vi "Washer DOE SM.vi"() -> ()   [LabVIEW 2012]
uses:
  Nufi/subVI/States.ctl
  Nufi/subVI/Data.ctl
  Nufi/subVI/logData.ctl
  C:/Users/220038920/Desktop/CVS Folder/NI-2010/Trunk/Washer DOE/Portable Stand/Nufi/dll/GeaCommunication.dll
  Nufi/dll/GeaCommunication.dll
  Nufi/subVI/Nufi Global_ReceivedDataCluster.vi
  <vilib>/Utility/file.llb/Read From Spreadsheet File (string).vi
panel:
  out "Model Information":string[][](array[string])
  out "Elapsed Time (sec)":dbl format="%.2f"
  out "Current State":string
  in  "First Time Through":bool=TRUE
  out "error out":errorcluster
  in  "Total Gallons Hot":dbl
  in  "Total Gallons Cold":dbl
  out "Loop Time":dbl
  in  "FrontPanel Meters 2":T1
  in  "Tab Control":enum32{"Test Screen", "Raw Data"}(tab)
  in  "Tab Control 3":T2(tab)
  in  "Initial Cloth Weight":dbl
  out "Enter File Init State":bool
  out "All Fields Complete":bool
  in  "Agitator:":u16(ring) items=["", "YES", "NO"]
  in  "File Setup OK":bool
  in  "Comments:":string
  in  "Voltage:":dbl
  in  "Water Pressure:":dbl
  in  "Cycle Selection:":string
  in  "Cold Water Temperature (Fahrenheit):":string
  in  "Hot Water Temperature (Fahrenheit):":string
  in  "Cloth Lot:":string
  in  "Capacity (cu.ft):":dbl
  in  "Hot Rinse Available:":u16(ring)
  in  "Extra Hot Wash Available:":u16(ring)
  in  "Number of Warm Washes:":dbl
  in  "Fill Method:":string
  in  "Station ID:":u16(ring) items=["", "Station 1", "Station 2", "Station 3", "Station 4", "Station 5", "Station 6", "Station 7", "Station 8", ""]
  in  "Lab ID:":string
  out "Test Date:":timestamp
  in  "Serial Number:":string
  in  "Model Number:":string
  in  "Engineer:":string
  in  "Technician:":string
  in  "Engineering ID:":string
  in  "Special Notes:":string
  out "File Path":path
  out "Complete?":bool
  in  "Update Button":bool
  in  "Manual Fill":bool
  in  "Coin Op":bool
  in  "Hawk":bool
  in  "Viper":bool
  in  "Complete DOE Cap":bool
  in  "Washer 4":T3
  in  "Washer 3":T4
  in  "Washer 2":T5
  in  "Washer 1":T6
  out "Test Date:DOE Cap":timestamp caption="Test Date:"
  out "Technician:DOE Cap":string caption="Technician:"
  in  "Command:Data":string caption="Debug Log"
  in  "Clear":bool
  in  "StartLog":bool
  in  "Path":bool
  out "UI Version":string
  out "Param. Ver.":string
  out "Personality":string
  in  "recirc":bool
  out "Recirc":bool
  in  "drain":bool
  out "Drain":bool
  in  "fs":bool
  out "FS":bool
  in  "det":bool
  out "Det":bool
  in  "cold":bool
  out "Cold":bool
  in  "hot":bool
  out "Hot":bool
  in  "Viper/Hawk":u16(ring) items=["Viper", "Hawk"]
  in  "Source":u8=228 format="%x"
  in  "Address":u8=35 format="%x"
  out "GEA2":bool
  out "Board ID":string
  out "Lid Closed?":bool
  out "Lid Locked?":bool
  out "FrontPanel Meters":T7 {"Rinse Hot" format="%#.3g"; "Rinse Cold" format="%#.3g"; "Hot Water Total During Wash" format="%#.3g"; "Cold Water Total During Wash" format="%#.3g"; "Volts" format="%#.3g"; "Current" format="%#.3g"; "Watts" format="%#.3g"; "Watt Hour" format="%#.3g"; "Hot Water Total" format="%#.3g"; "Hot Water Rate" format="%#.3g"; "Cold Water Total" format="%#.3g"; "Cold Water Rate" format="%#.3g"; "Hot Water Pressure" format="%#.3g"; "Hot Water Temperature" format="%#.3g"; "Cold Water Pressure" format="%#.3g"; "Cold Water Temperature" format="%#.3g"}
  out "Fabric Softener":u32
  out "Detergent":u32
  out "Speed":u32
  out "Load Size":u32
  out "Direction":string
  out "Temperature":u8
  out "Water Pressure":u32
  in  "Off Mode Watts":dbl
  in  "Standby Mode Watts":dbl
  out "Elapsed Time":dbl format="%<%H:%M:%S>t"
  in  "Tab Control 4":enum32{"Watts", "Control Settings"}(tab)
  out "Recirc 3":dbl(graph)
  out "Incoder Position":string
  out "Pre Soak":string
  out "Spin Setting":string
  out "Temperature Setting":string
  out "Soil Setting":string
  out "Total Gallons Used":string
  in  "Stop":bool
  in  "Start":bool
  in  "Reset All":bool
  out "Array":string[][](array[string])
  in  "DOE Capacity Path":path=path "C:/GE/Washer DOE/DOE Capacity.txt"
  in  "Calibration File Path":path=path "C:/Program Files/GE/Washer DOE/CalibrationDates.txt"
  in  "VISA Laurel Meter":refnum<visa-resource-name>="LaurelMeter"
  in  "Aplus IP Address":string="192.168.1.101"
  in  "Remote Port":i32=502
  out "Start Time (sec)":dbl format="%<%H:%M:%S>t"
  in  "Send":bool
  in  "Data":u8[](array[numeric]) format="%.0x"
  in  "Command":u8 format="%.0x"
  in  "Exit":bool
  in  "EOL":bool
  in  "2015?":bool
  in  "Low Power Switch":bool
  in  "SaveGraph":bool
  in  "All Models Excel Sheet":path=path "C:/GE/Washer DOE"
  in  "Network Model Location":path=path "\\\\3.67.38.12\\share/Test Data/Washer DOE/Models"
  # "Take the Family, Model, and Capacity."
  # "Test Conditions"
  # "Model Details"
  # "DOE Capacity Measurements Per 10 CFR 430 Appendix J1"
  # "Standard Values"
  # "Measured\nTemp (Deg F)"
  # "Weigh of \nWater (lbs)"
  # "Model Number"
  # "Serial Number"
  # "Lab Number"
  # "This will only update at the end of the cycle"
  # "x"
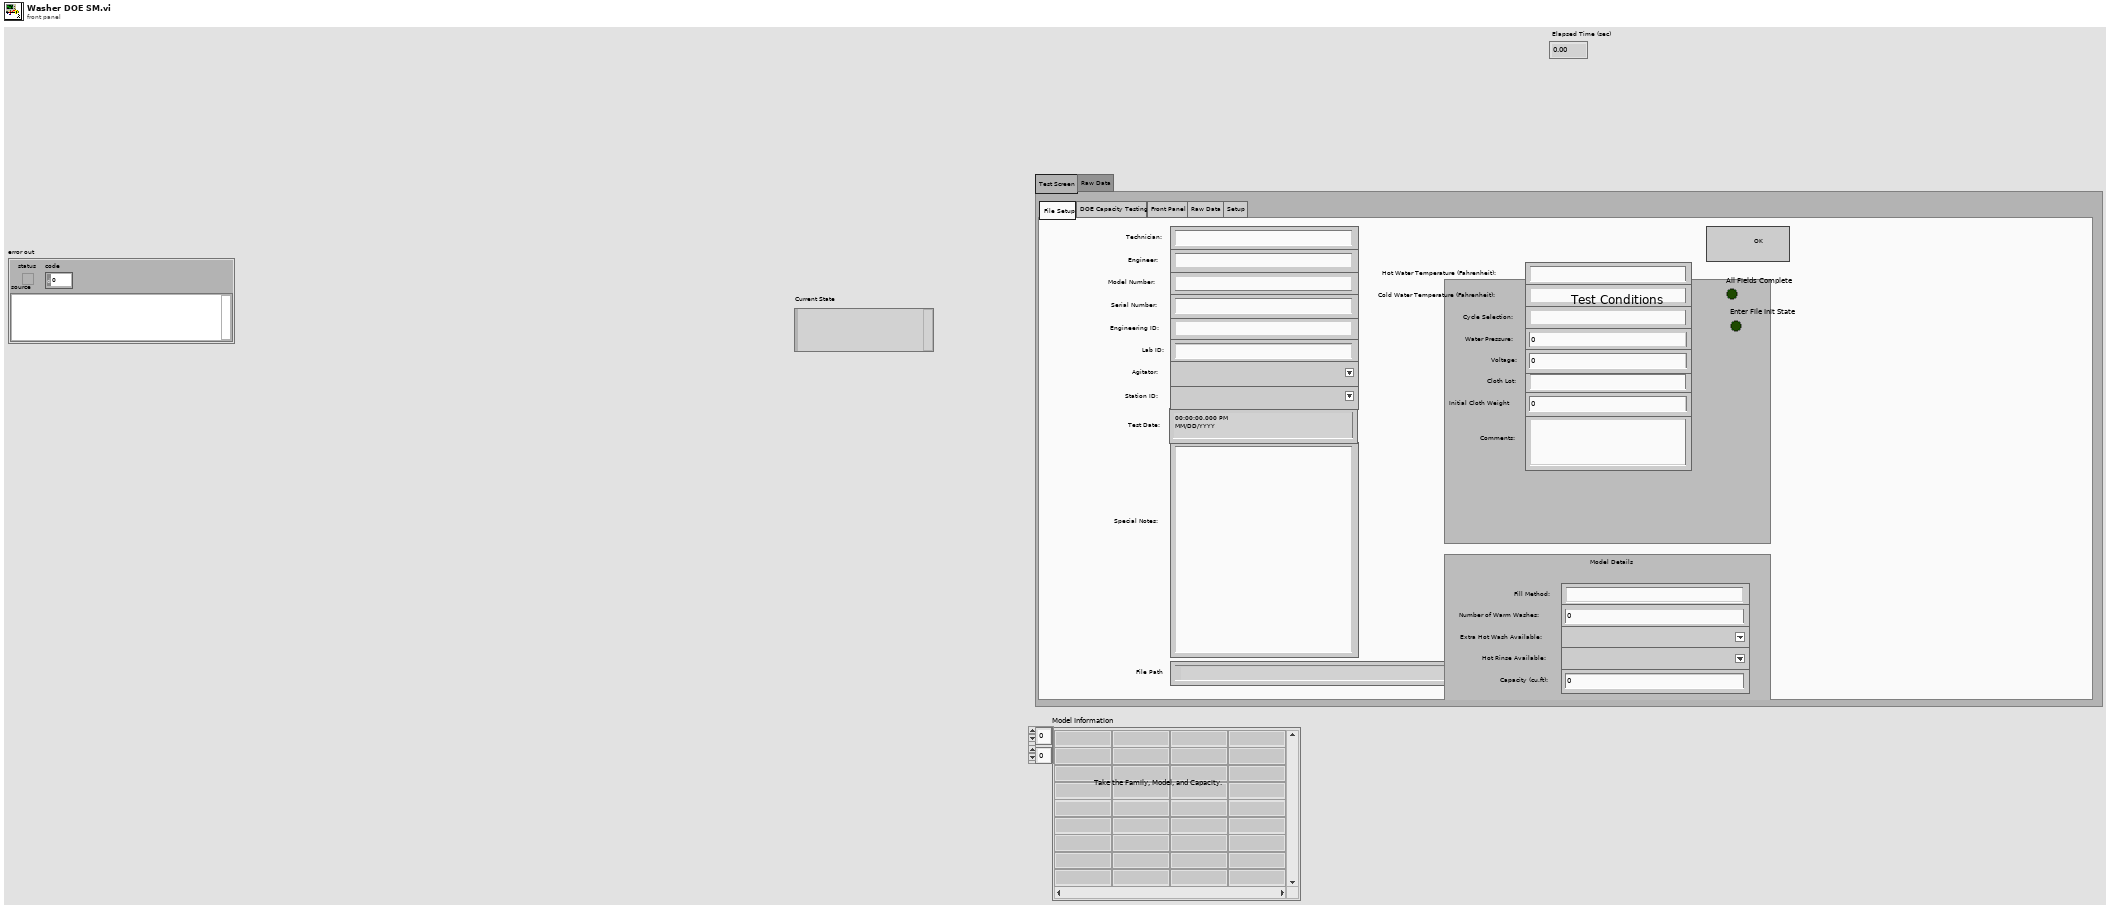
[diagram p1: front panel]
types:
  T1 = cluster{"Cold Water\nTemperature":dbl, "Cold Water\nPressure":dbl, "Hot Water\nTemperature":dbl, "Hot Water\nPressure":dbl, "Cold Water\nRate":dbl, "Cold Water\nTotal":dbl, "Hot Water\n Rate":dbl, "Hot Water\nTotal":dbl, "Watt Hour":dbl, "Watts":dbl, "Current":dbl, "Volts":dbl, "Cold Water Total During Wash":dbl, "Hot Water Total During Wash":dbl, "Rinse Cold":dbl, "Rinse Hot":dbl}
  T2 = enum32{"File Setup", "DOE Capacity Testing", "Front Panel", "Raw Data", "Setup"}
  T3 = cluster{"Measured Temp (Deg F)3":dbl, "Weight of Water (lbs)3":dbl, "Lab Number3":string, "Serial Number3":string, "Model Number3":string}
  T4 = cluster{"Measured Temp (Deg F)2":dbl, "Weight of Water (lbs)2":dbl, "Lab Number2":string, "Serial Number2":string, "Model Number2":string}
  T5 = cluster{"Measured Temp (Deg F )1":dbl, "Weight of Water (lbs)1":dbl, "Lab Number1":string, "Serial Number1":string, "Model Number1":string}
  T6 = cluster{"Measured Temp":dbl, "Water Weight":dbl, "Lab Number":string, "Serial Number":string, "Model Number":string}
  T7 = cluster{"Cold Water Temperature":dbl, "Cold Water Pressure":dbl, "Hot Water Temperature":dbl, "Hot Water Pressure":dbl, "Cold Water Rate":dbl, "Cold Water Total":dbl, "Hot Water Rate":dbl, "Hot Water Total":dbl, "Watt Hour":dbl, "Watts":dbl, "Current":dbl, "Volts":dbl, "Cold Water Total During Wash":dbl, "Hot Water Total During Wash":dbl, "Rinse Cold":dbl, "Rinse Hot":dbl}
  T8 = typedef "Data.ctl" = cluster{"GEA2 Message Ref":refnum<k24>, "Board ID":string, "USB Connect":refnum<k24>, "GEA Bus":refnum<k24>, "Address":u8, "Source":u8, "Message Count":dbl, "ReceivedData":u8[], "Log?":bool, "Partial Message String":string, "Full Message to Save":string, "Data to send":u8[], "Command":u8, "selected path":path, "debugRef":refnum<file>, "dataRef":refnum<file>, "logData":T9, "GraphData":T9[]}
  T9 = typedef "logData.ctl" = cluster{"IGBT Temp":u8, "Speed":u32, "Load Size":u32, "Temperature":u8, "Water Pressure":u32, "Detergent":u32, "Fabric Softener":u32, "Direction":string, "Det":bool, "FS":bool, "Recirc":bool, "Drain":bool, "Hot":bool, "Cold":bool, "LidClosed":bool, "LidLocked":bool}
  T10 = typedef "States.ctl" = enum16{"-------- Initialize --------", "Data", "GEA2", "---------- Core ----------", "Wait", "Read Debug", "Read MC Data", "Read Inv Data", "Read Incoder Position", "Read LEDs", "Update Graphs", "Send CMD", "Log Debug", "Log Data", "Test", "Exit"}
  T11 = enum8{"Enabled", "Disabled", "Disabled and Grayed Out"}
  T12 = typedef "Nufi Message.ctl" = cluster{"ReceivedData":u8[], "Count":dbl, "Source Address":u8, "Destination Addresss":u8, "Command":u8, "Days":i32, "Hours":i32, "Minutes":i32, "Seconds":i32, "Milliseconds":i32}
  T13 = enum16{"open", "replace", "create", "open or create", "replace or create", "replace or create with confirmation"}
  T14 = cluster{"IGBT Temp":bool, "Speed":bool, "Load Size":bool, "Temperature":bool, "Water Pressure":bool, "Detergent":bool, "Fabric Softener":bool, "Direction":bool, "Det":bool, "FS":bool, "Recirc":bool, "Drain":bool, "Hot":bool, "Cold":bool, "LidClosed":bool, "LidLocked":bool}
  T15 = enum32{"invalid app kind", "Development System", "Run Time System", "Student Edition", "Embedded LabVIEW", "Evaluation", "Custom"}
  T16 = enum16{"Command Mode", "Cold Reset", "Function Reset", "Reading: All Active Items", "Reading: Item 1", "Reading: Item 2", "Reading: Item 3"}
  T17 = enum32{"Invalid", "Standard", "Closed", "Hidden", "Minimized", "Maximized"}
  T18 = cluster{"Measured Temp":dbl, "Weight of Water":dbl, "Lab Number":string, "Serial Number":string, "Model Number":string}
  T19 = cluster{"Core":cluster{"Current VI Reference":refnum<vi>, "Close Panel on Exit?":bool}, "Remote Port":i32, "Aplus IP Address":string, "Power":cluster{"Voltage":sgl, "Current":sgl, "Frequency":sgl, "Power":sgl, "Power Factor":sgl}, "Watt Hours":dbl, "Total Array":dbl[], "VISA Laurel Meter":refnum<visa-resource-name>, "FrontPanel Meters 2":cluster{"Cold Water\nTemperature":dbl, "Cold Water\nPressure":dbl, "Hot Water\nTemperature":dbl, "Hot Water\nPressure":dbl, "Cold Water\nRate":dbl, "Cold Water\nTotal":dbl, "Hot Water\n Rate":dbl, "Hot Water\nTotal":dbl, "Watt Hour":dbl, "Watts":dbl, "Current":dbl, "Volts":dbl, "Cold Water Total During Wash":dbl, "Hot Water Total During Wash":dbl, "Rinse Cold":dbl, "Rinse Hot":dbl}, "Total Gallons Cold":dbl, "Total Gallons Hot":dbl, "2015?":bool, "Off Mode Watts":dbl, "Standby Mode Watts":dbl, "Low Power Switch":bool, "First Time Through":bool, "Calibration":string[][], "Washer 1":cluster{"Measured Temp":dbl, "Water Weight":dbl, "Lab Number":string, "Serial Number":string, "Model Number":string}, "Washer 2":cluster{"Measured Temp (Deg F )1":dbl, "Weight of Water (lbs)1":dbl, "Lab Number1":string, "Serial Number1":string, "Model Number1":string}, "Washer 3":cluster{"Measured Temp (Deg F)2":dbl, "Weight of Water (lbs)2":dbl, "Lab Number2":string, "Serial Number2":string, "Model Number2":string}, "Washer 4":cluster{"Measured Temp (Deg F)3":dbl, "Weight of Water (lbs)3":dbl, "Lab Number3":string, "Serial Number3":string, "Model Number3":string}, cluster{"Calibration File Path":path, "DOE Capacity Path":path, "All Models Excel Sheet":path, "Network Model Location":path}, "Complete DOE Cap":bool}
  T20 = cluster{"Calibration File Path":path, "DOE Capacity Path":path, "All Models Excel Sheet":path, "Network Model Location":path}
  T21 = cluster{"Voltage":sgl, "Current":sgl, "Frequency":sgl, "Power":sgl, "Power Factor":sgl}
  T22 = cluster{"Current VI Reference":refnum<vi>, "Close Panel on Exit?":bool}
  T23 = cluster{"Cold Water Pressure":dbl, "Hot Water Pressure":dbl, "Cold Water Temp":dbl, "Hot Water Temp":dbl, "Ambient Temp":dbl, "Room Humidity":dbl}
  T24 = cluster{"Voltage":sgl, "Current":sgl, "Frequency":sgl, "Power":sgl, "Power Factor":sgl, "WattHours":sgl}
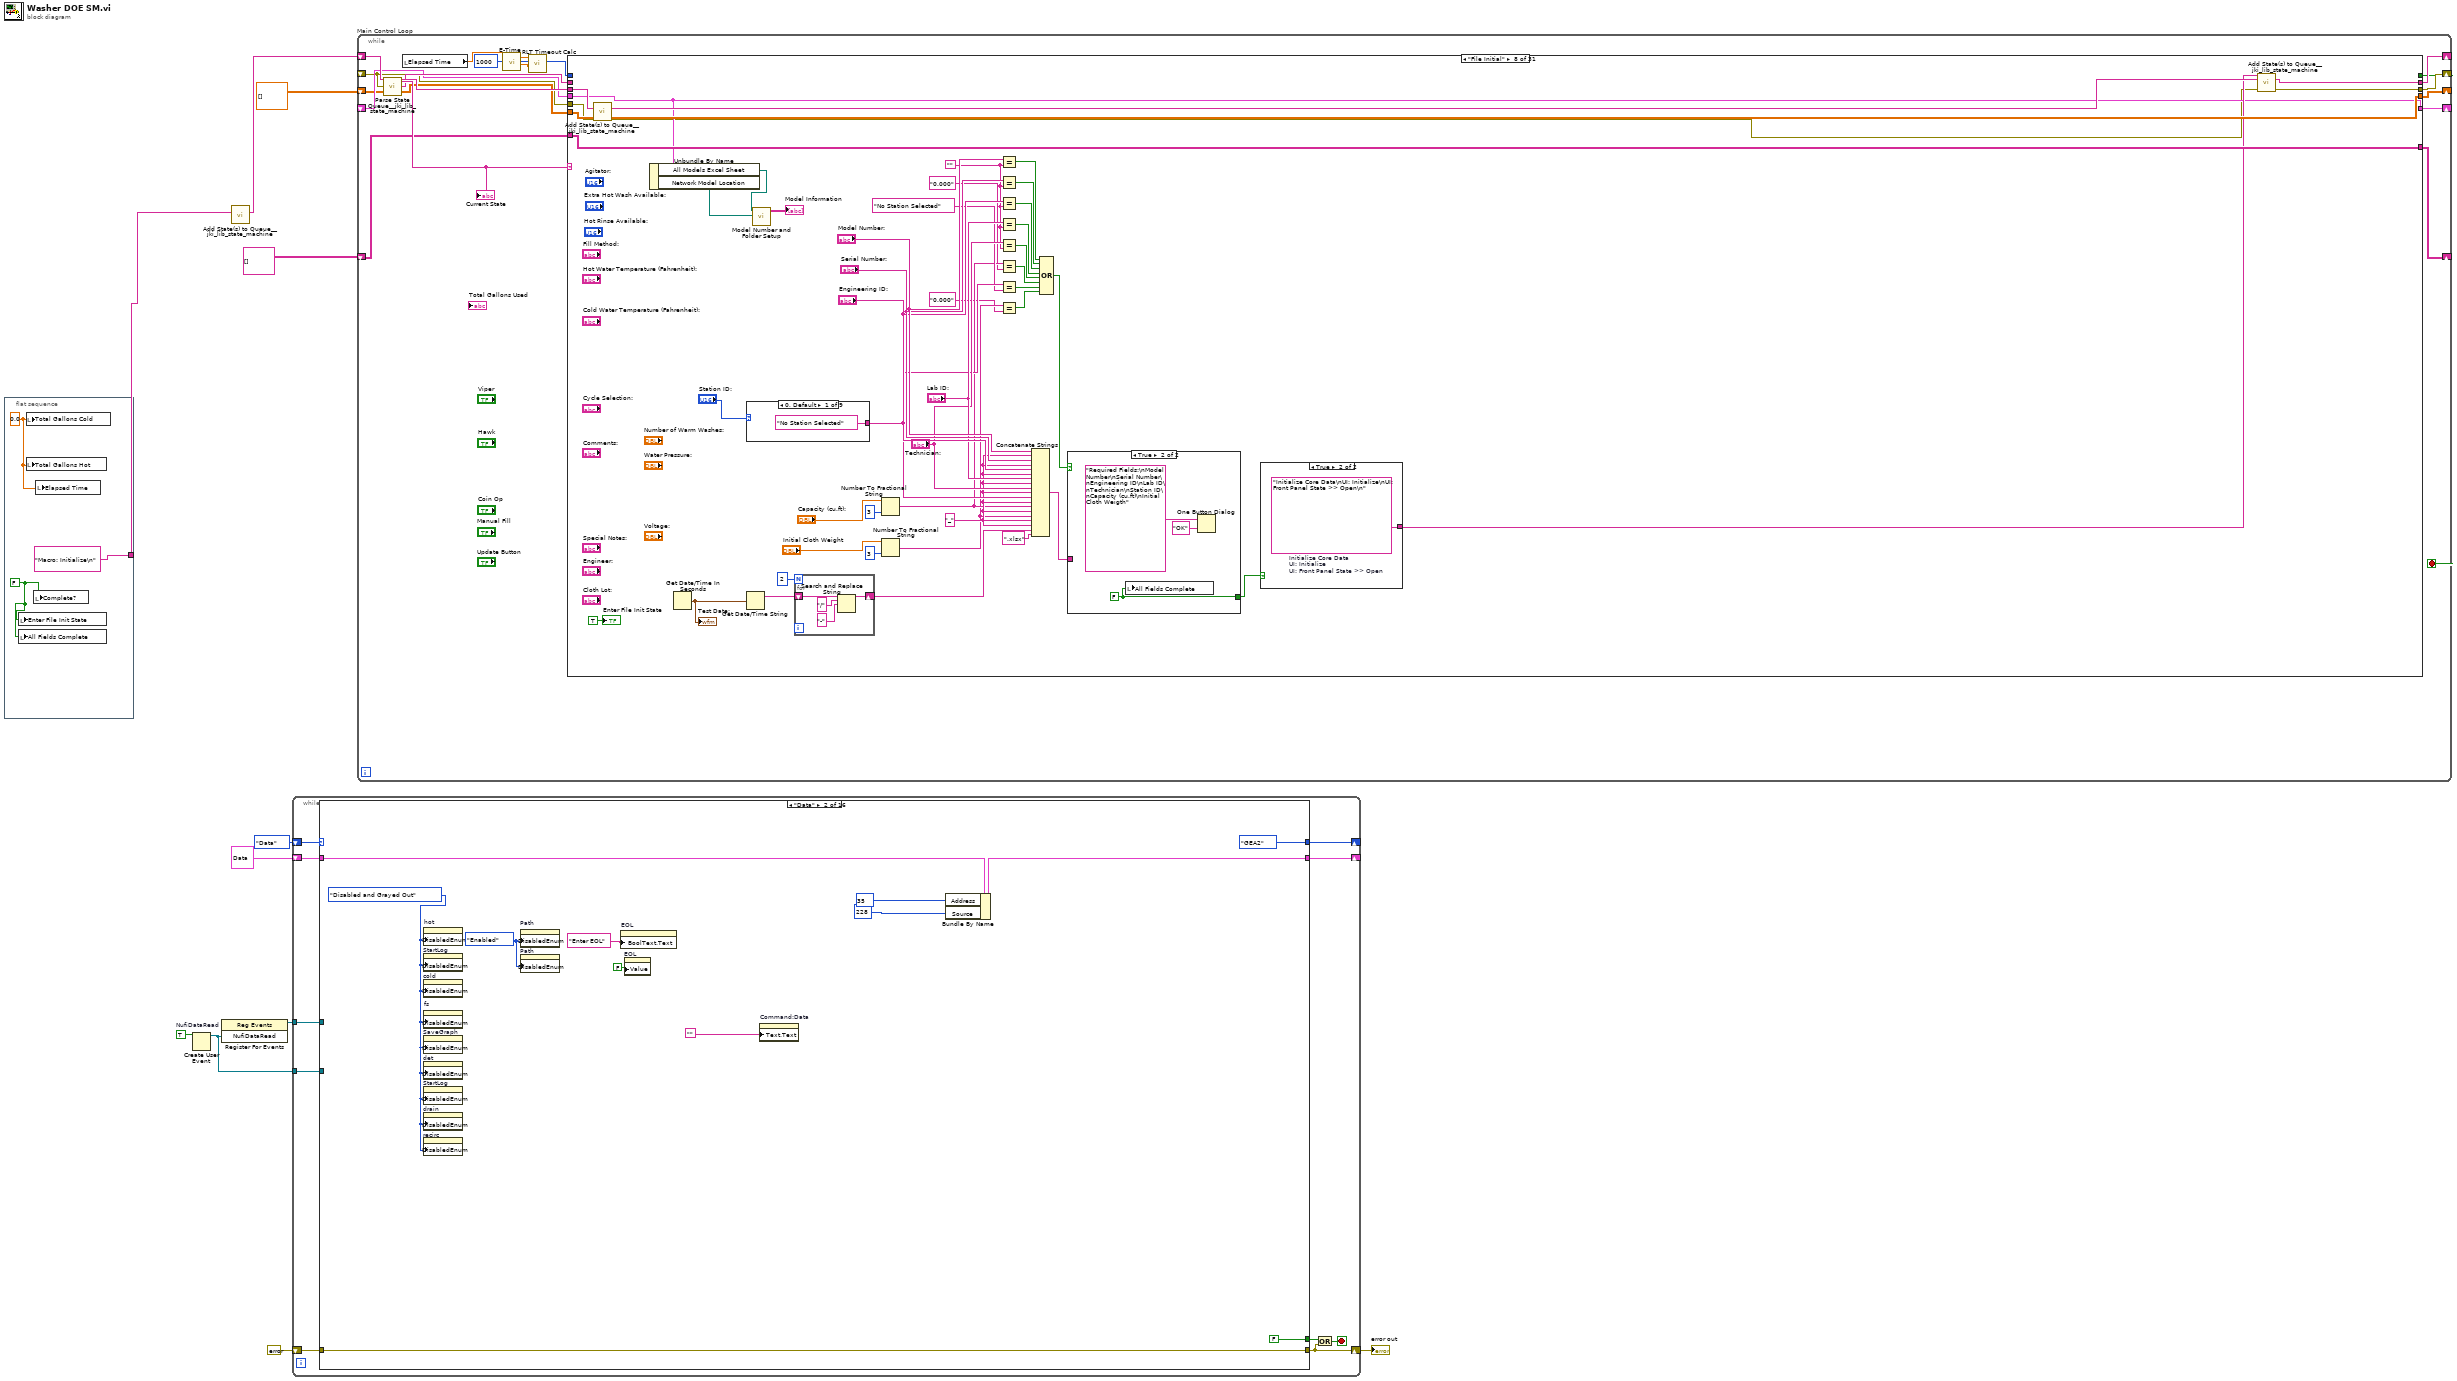
[diagram p0: block diagram]
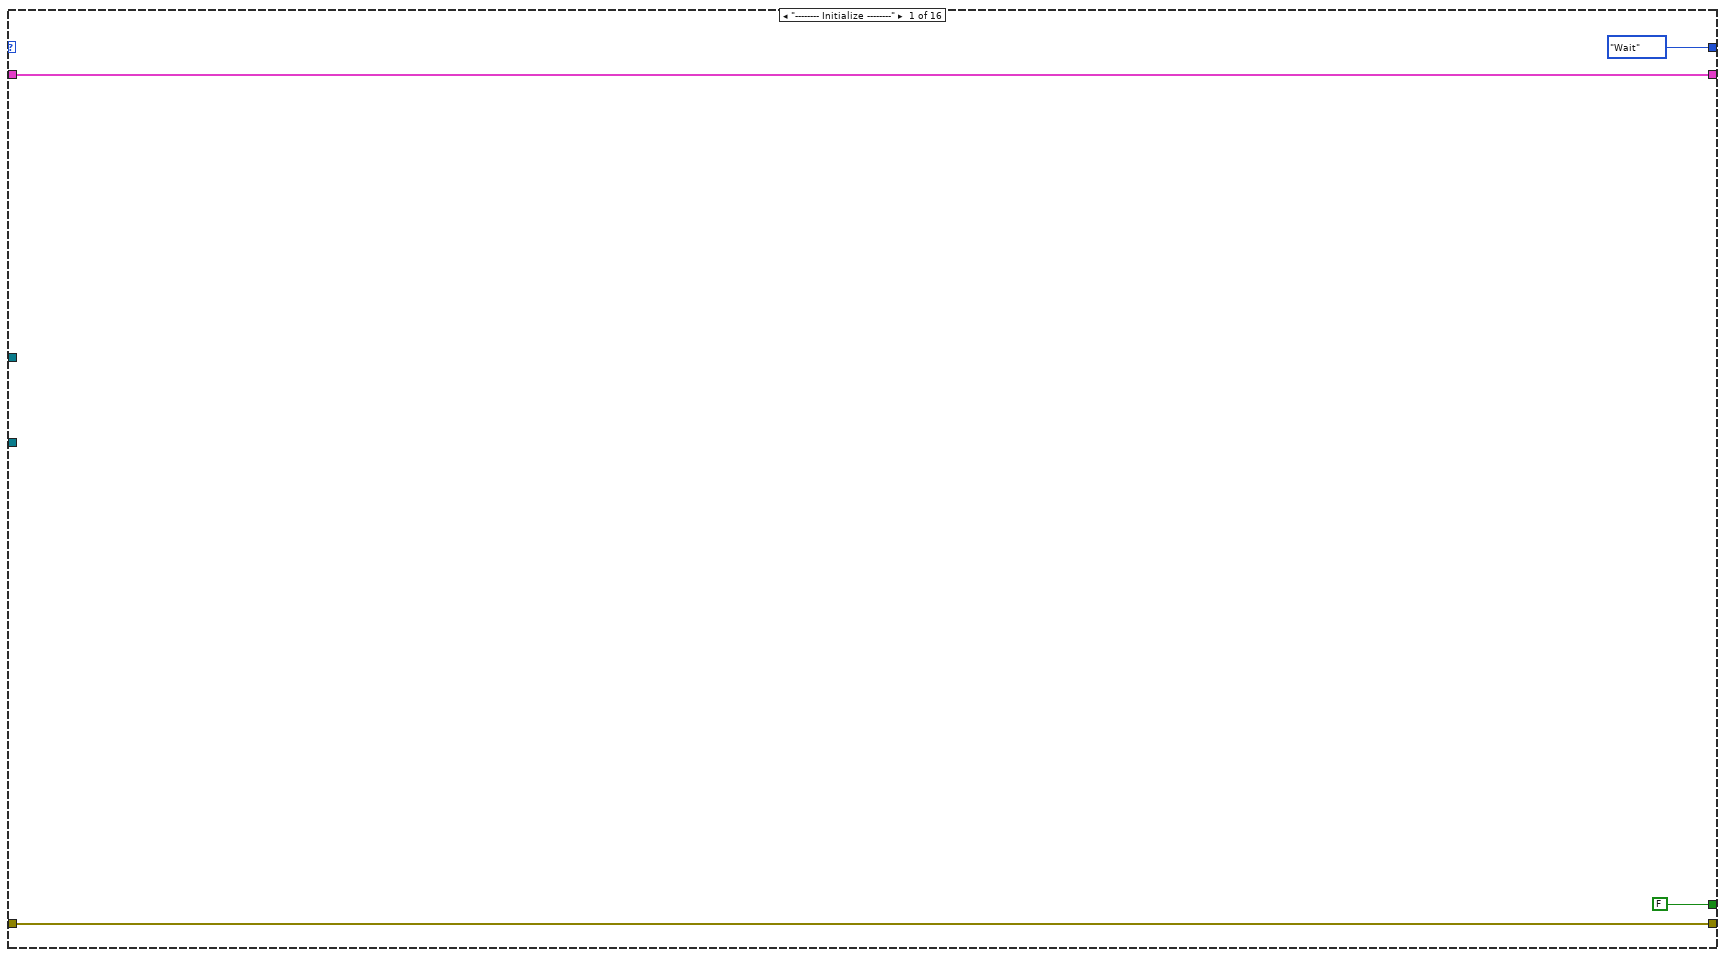
[diagram p2: hidden frame]
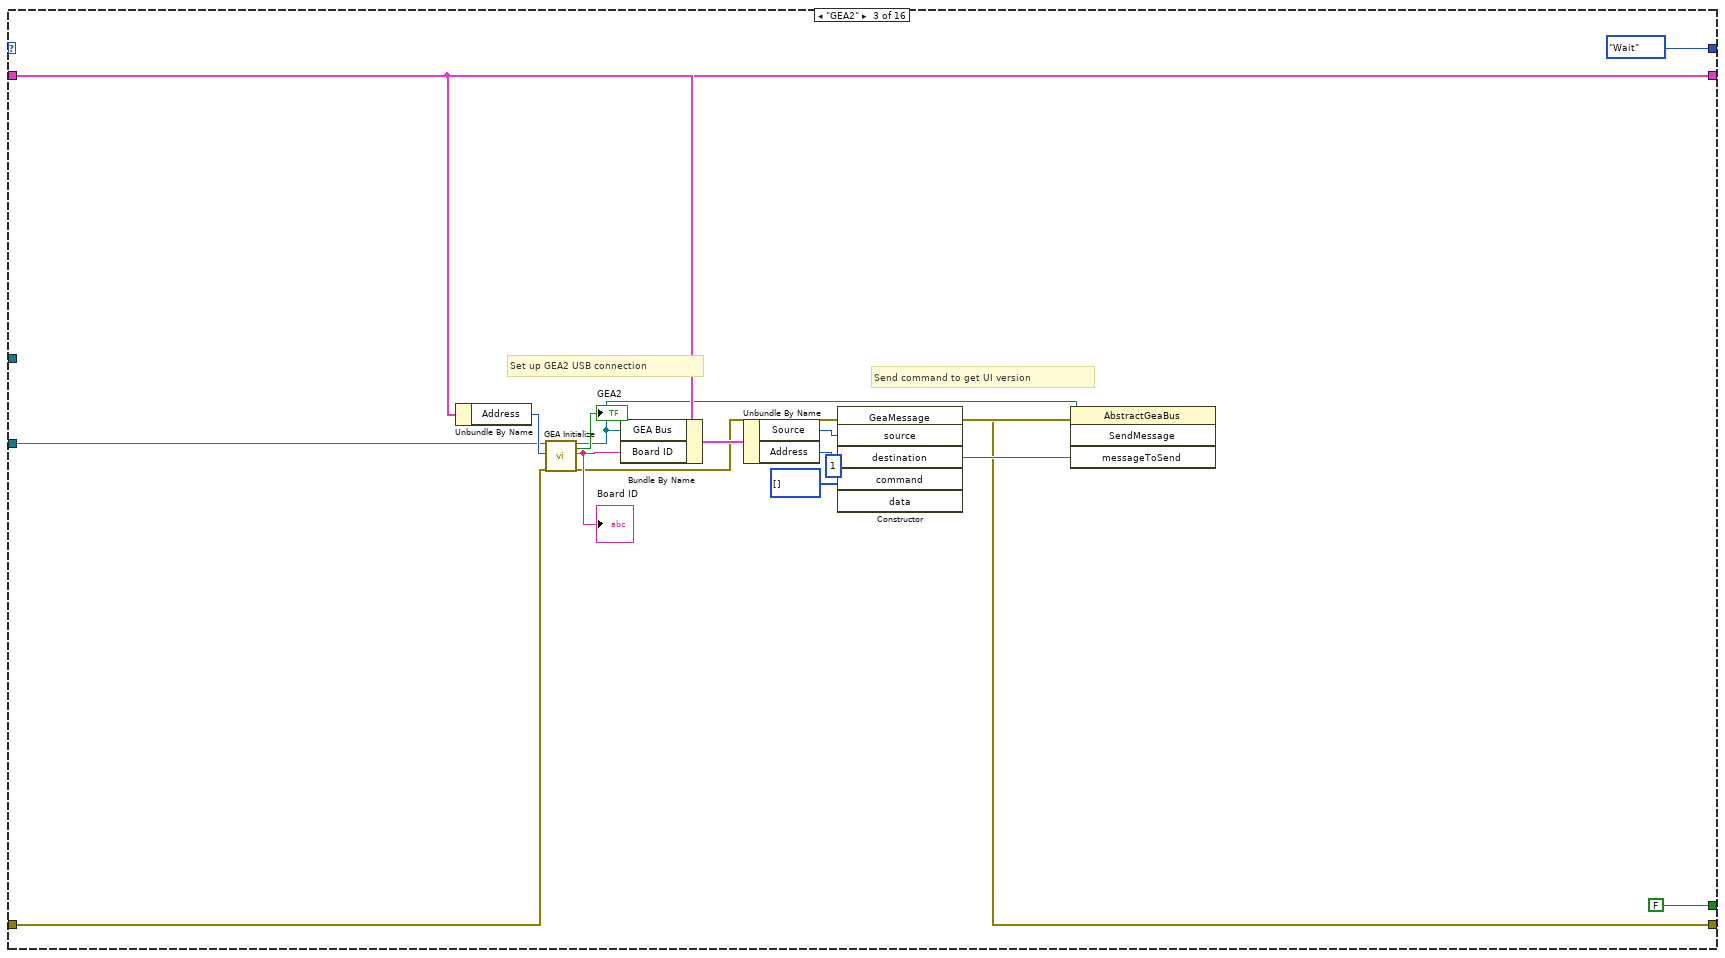
[diagram p3: hidden frame]
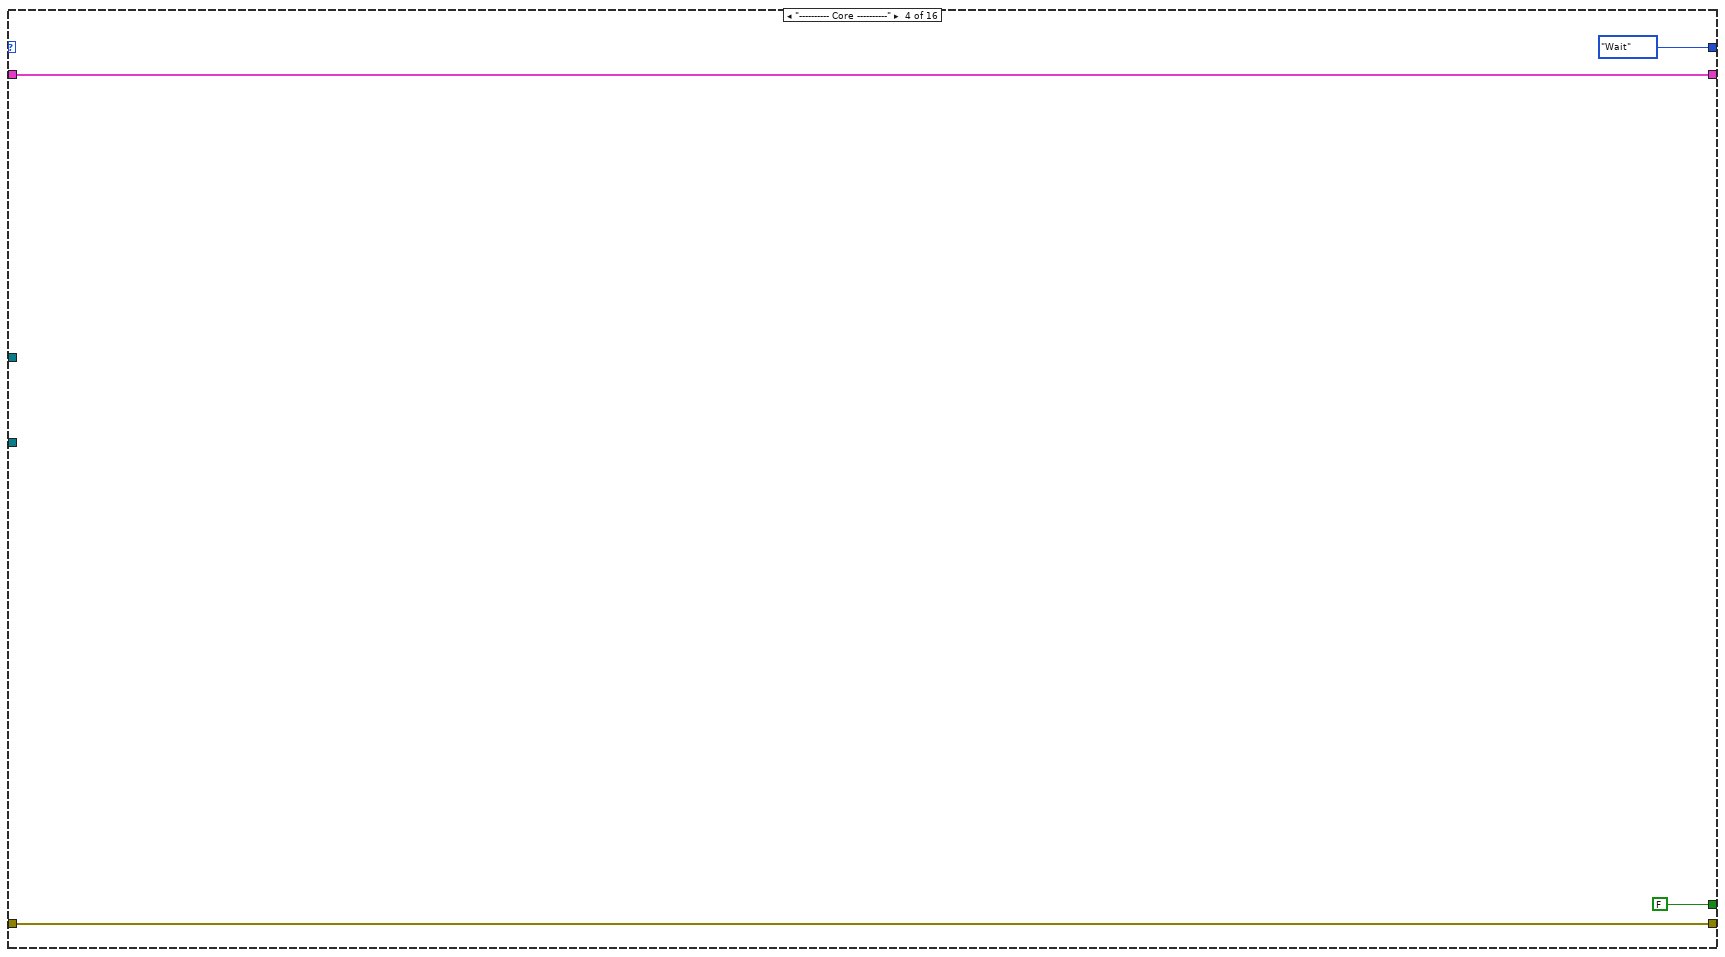
[diagram p4: hidden frame]
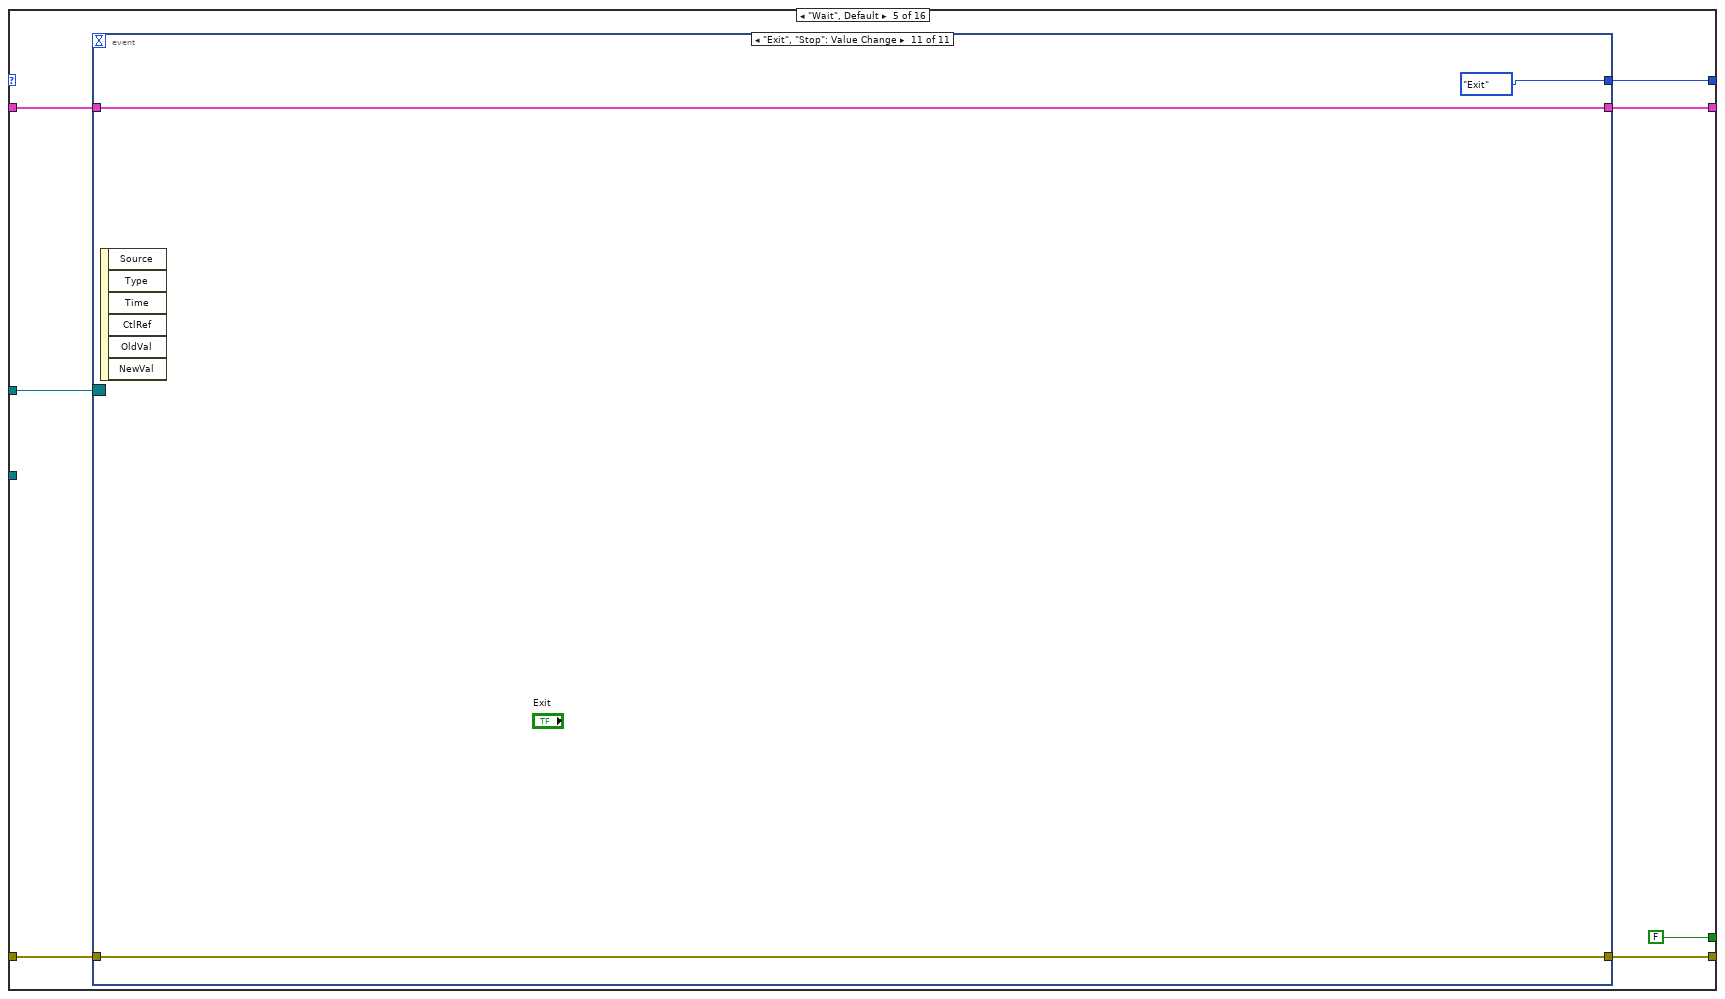
[diagram p5: hidden frame]
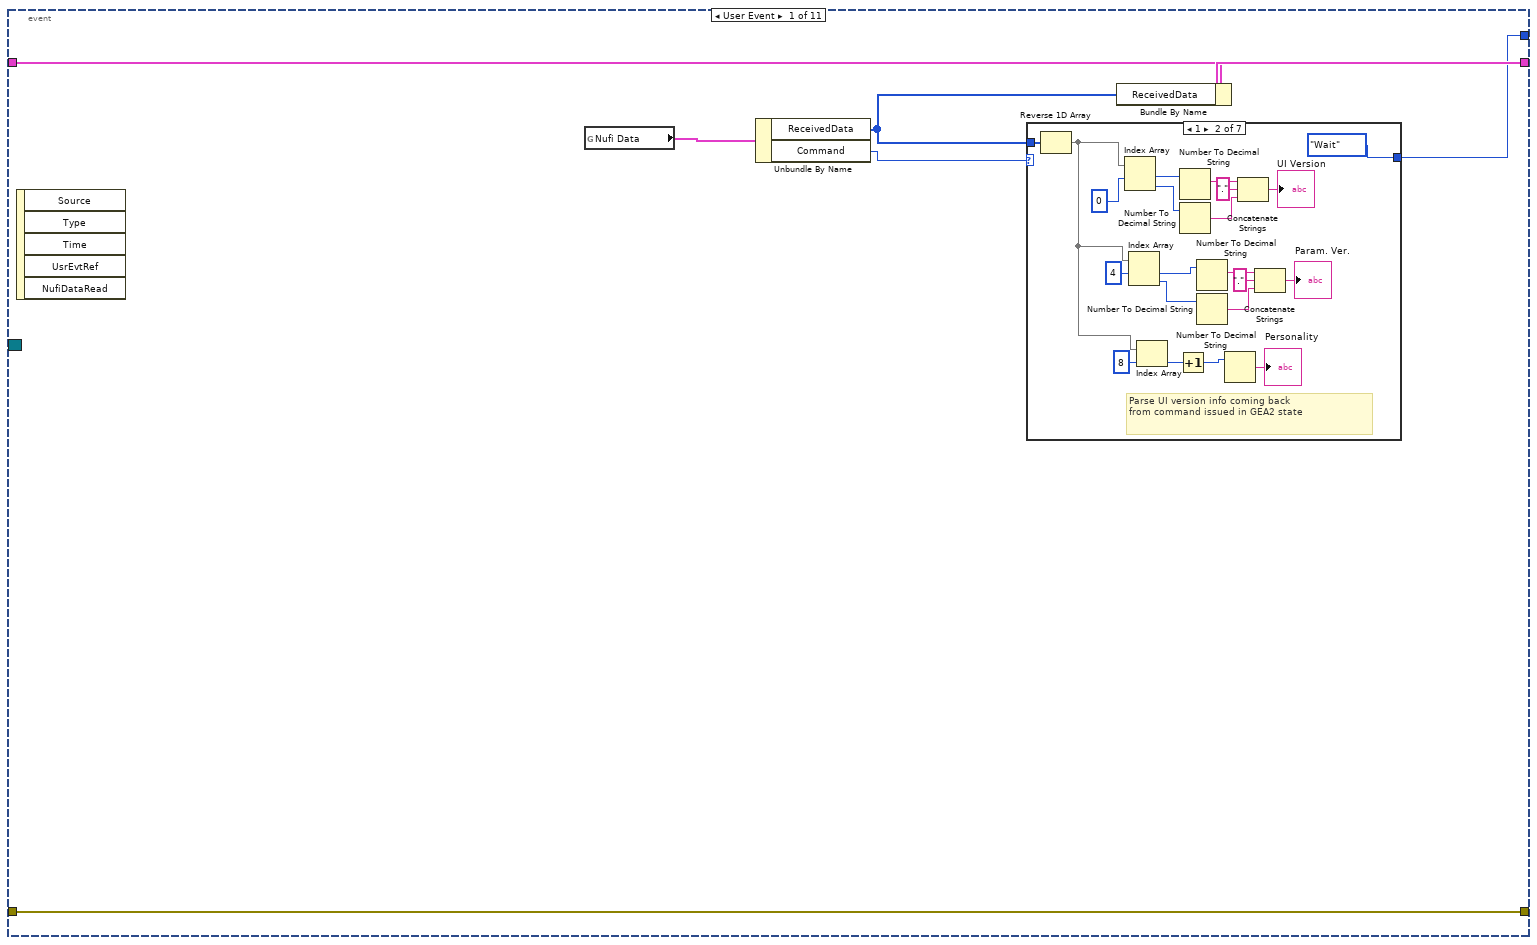
[diagram p6: hidden frame]
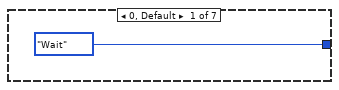
[diagram p7: hidden frame]
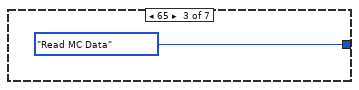
[diagram p8: hidden frame]
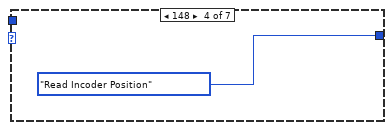
[diagram p9: hidden frame]
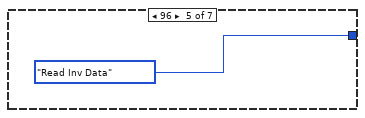
[diagram p10: hidden frame]
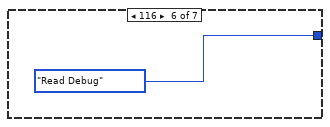
[diagram p11: hidden frame]
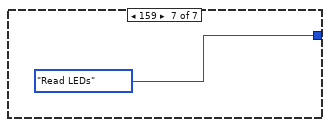
[diagram p12: hidden frame]
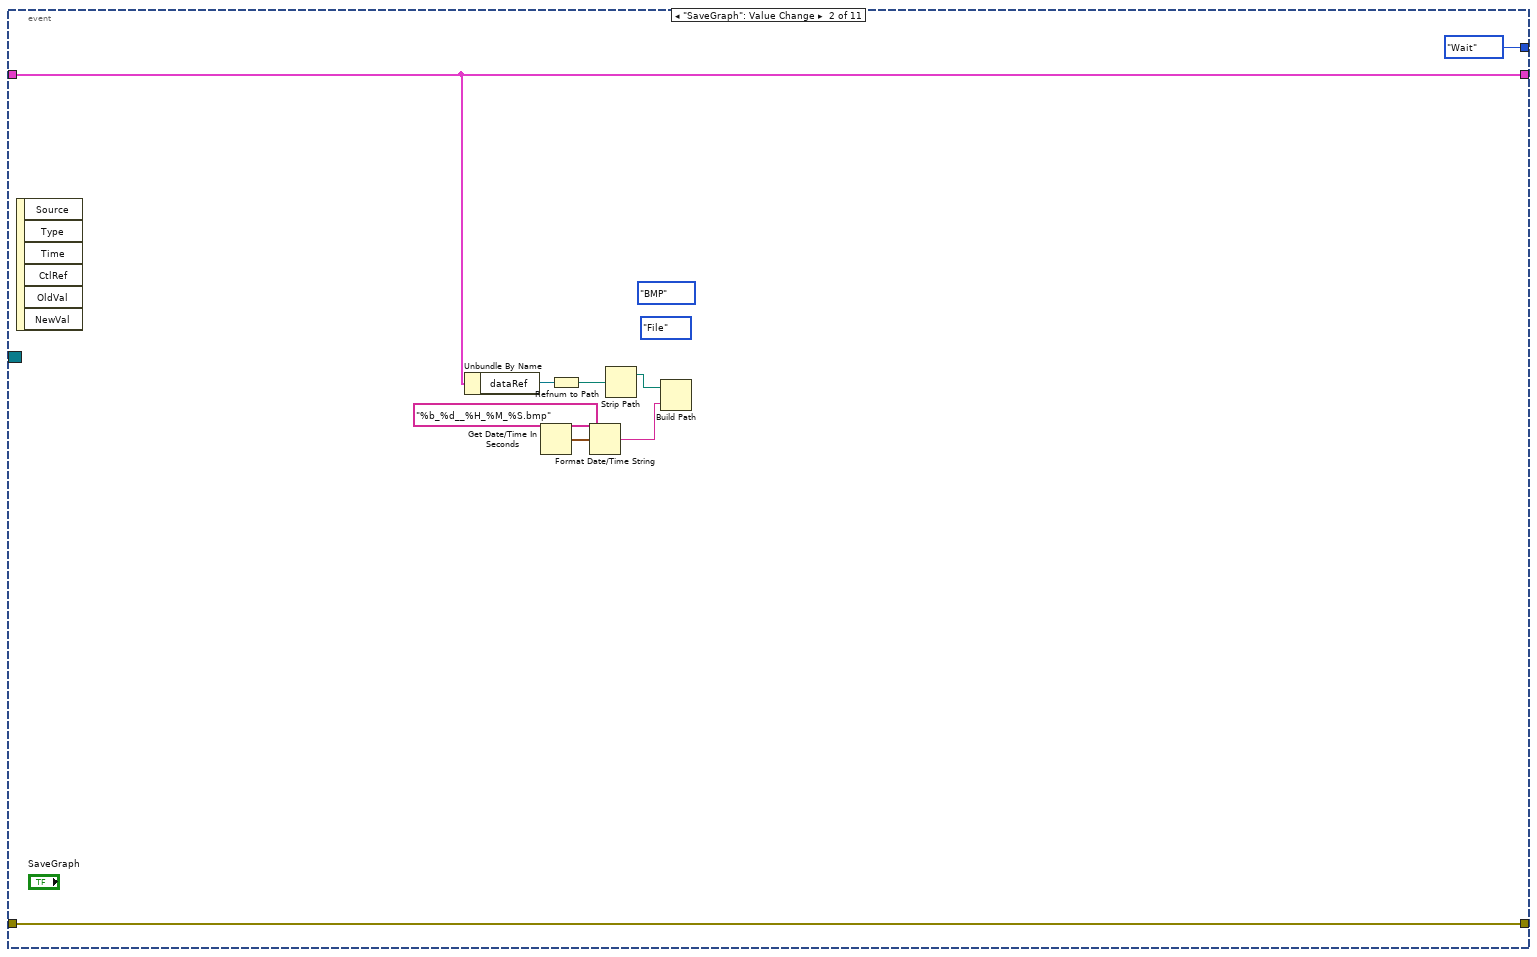
[diagram p13: hidden frame]
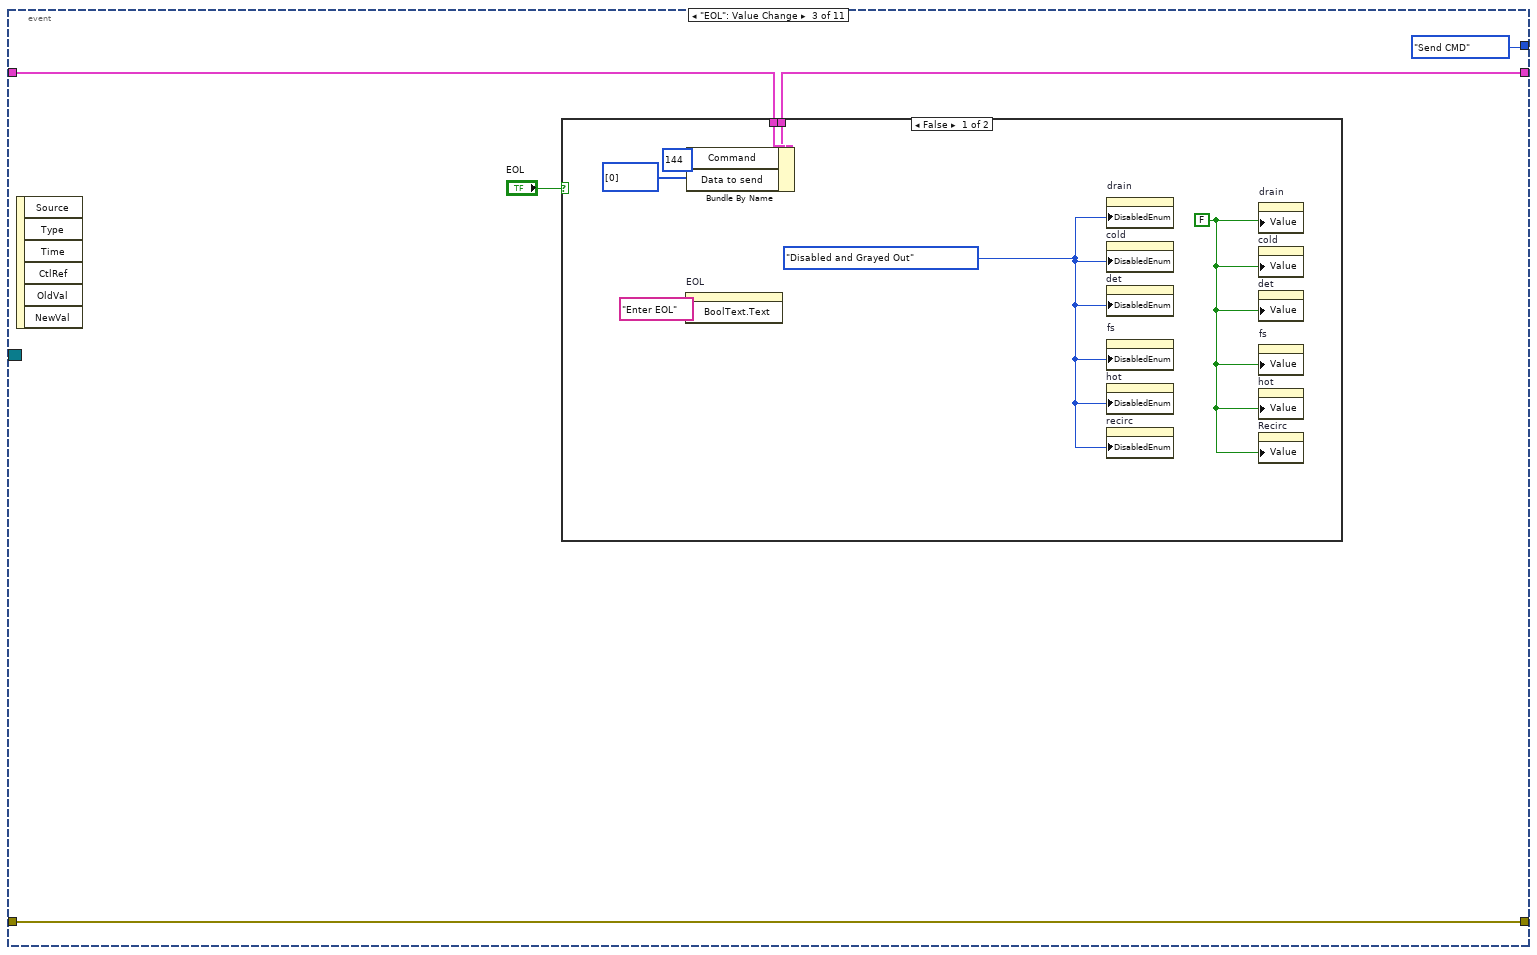
[diagram p14: hidden frame]
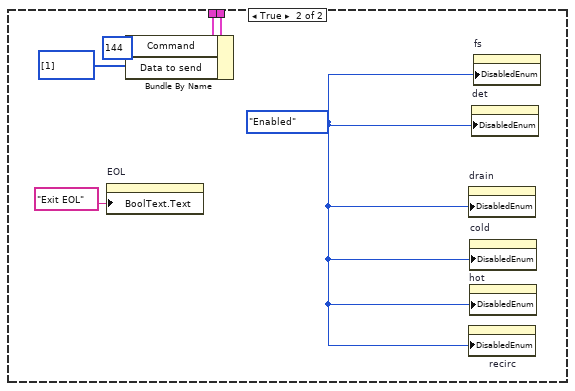
[diagram p15: hidden frame]
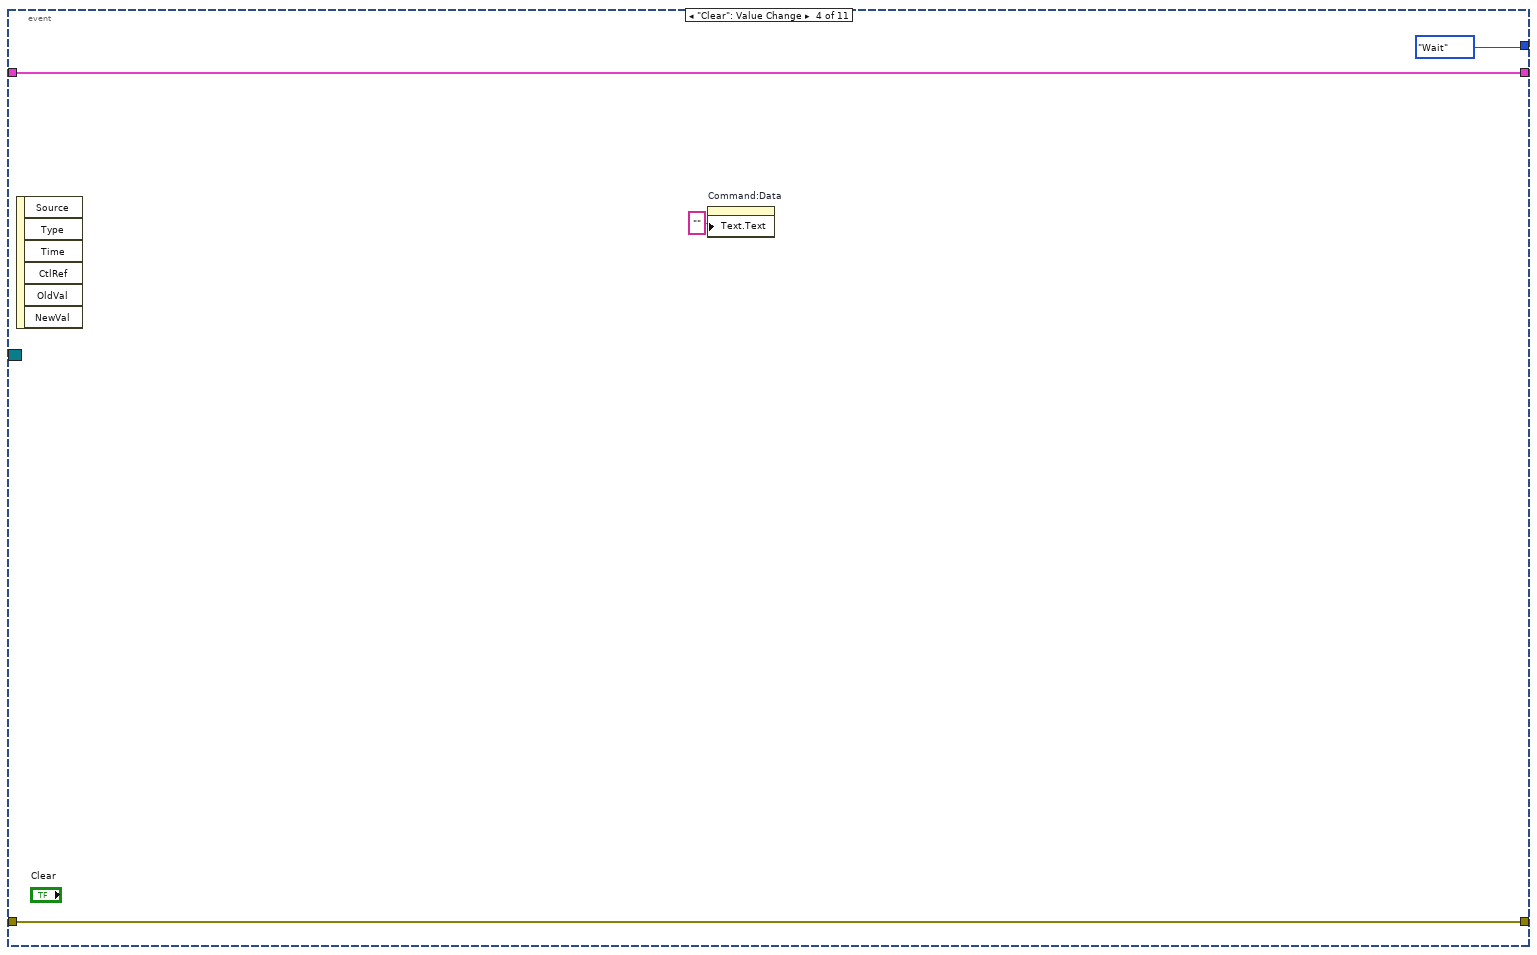
[diagram p16: hidden frame]
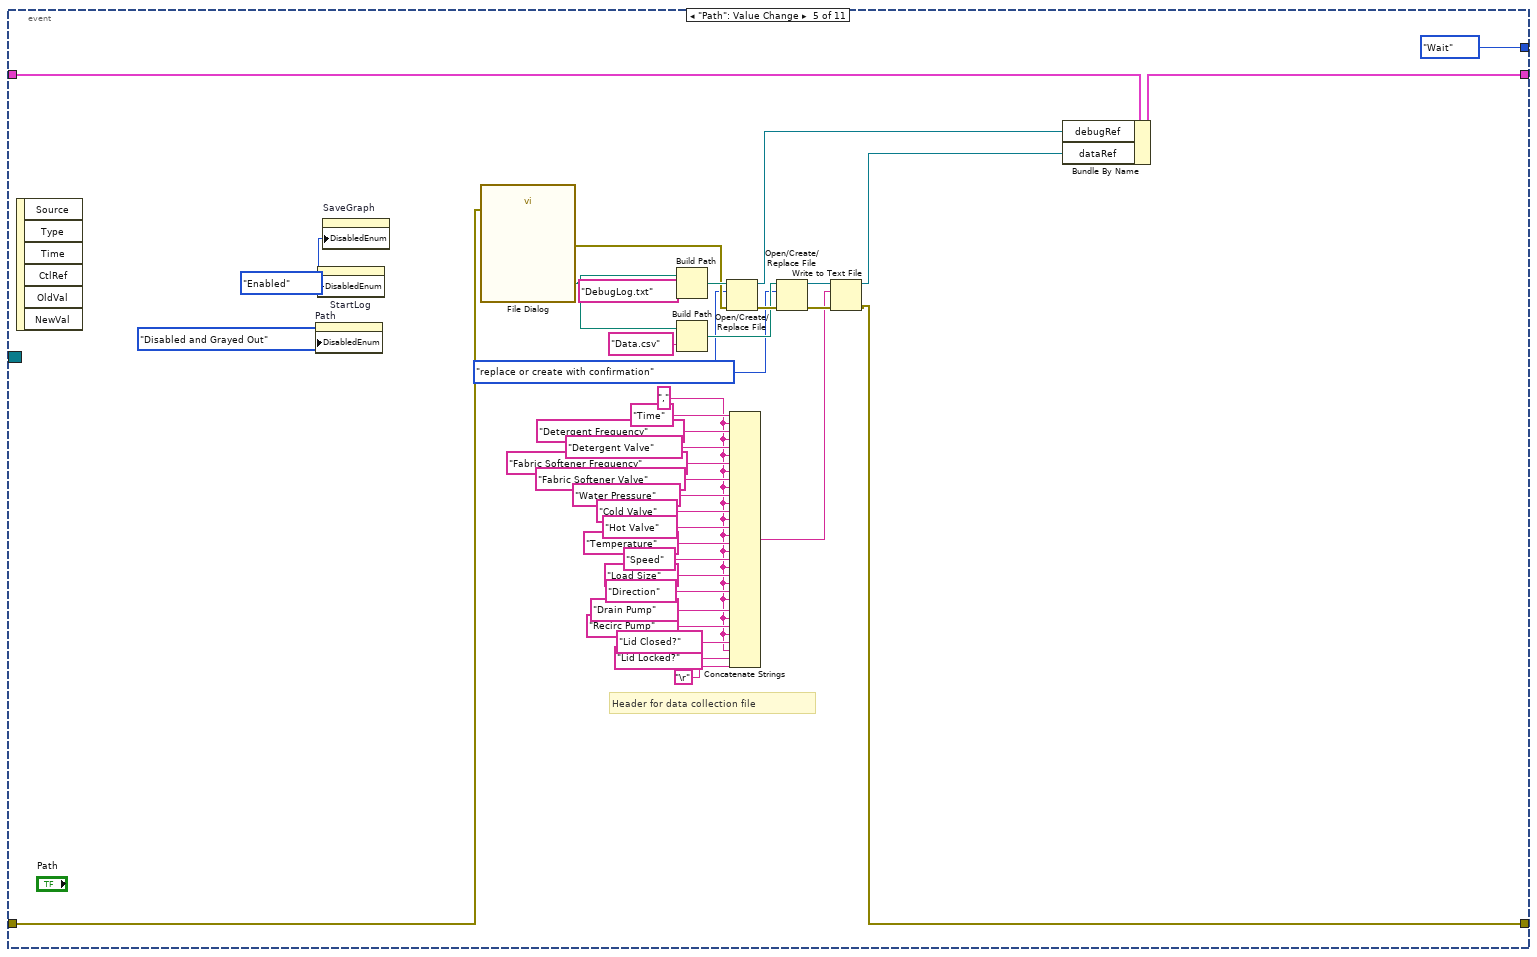
[diagram p17: hidden frame]
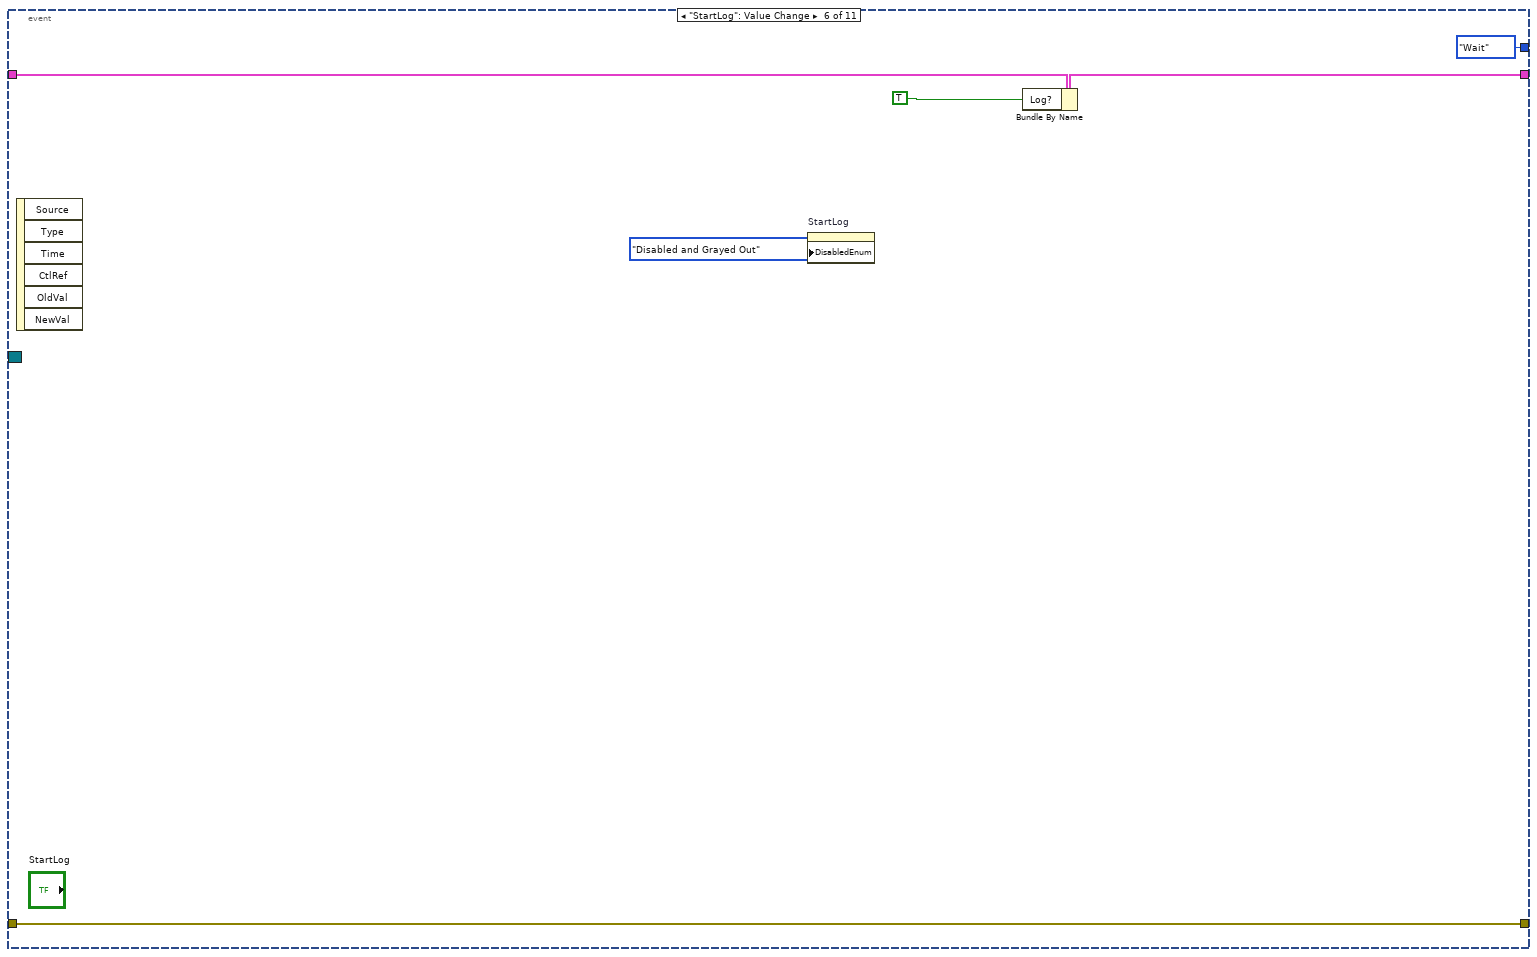
[diagram p18: hidden frame]
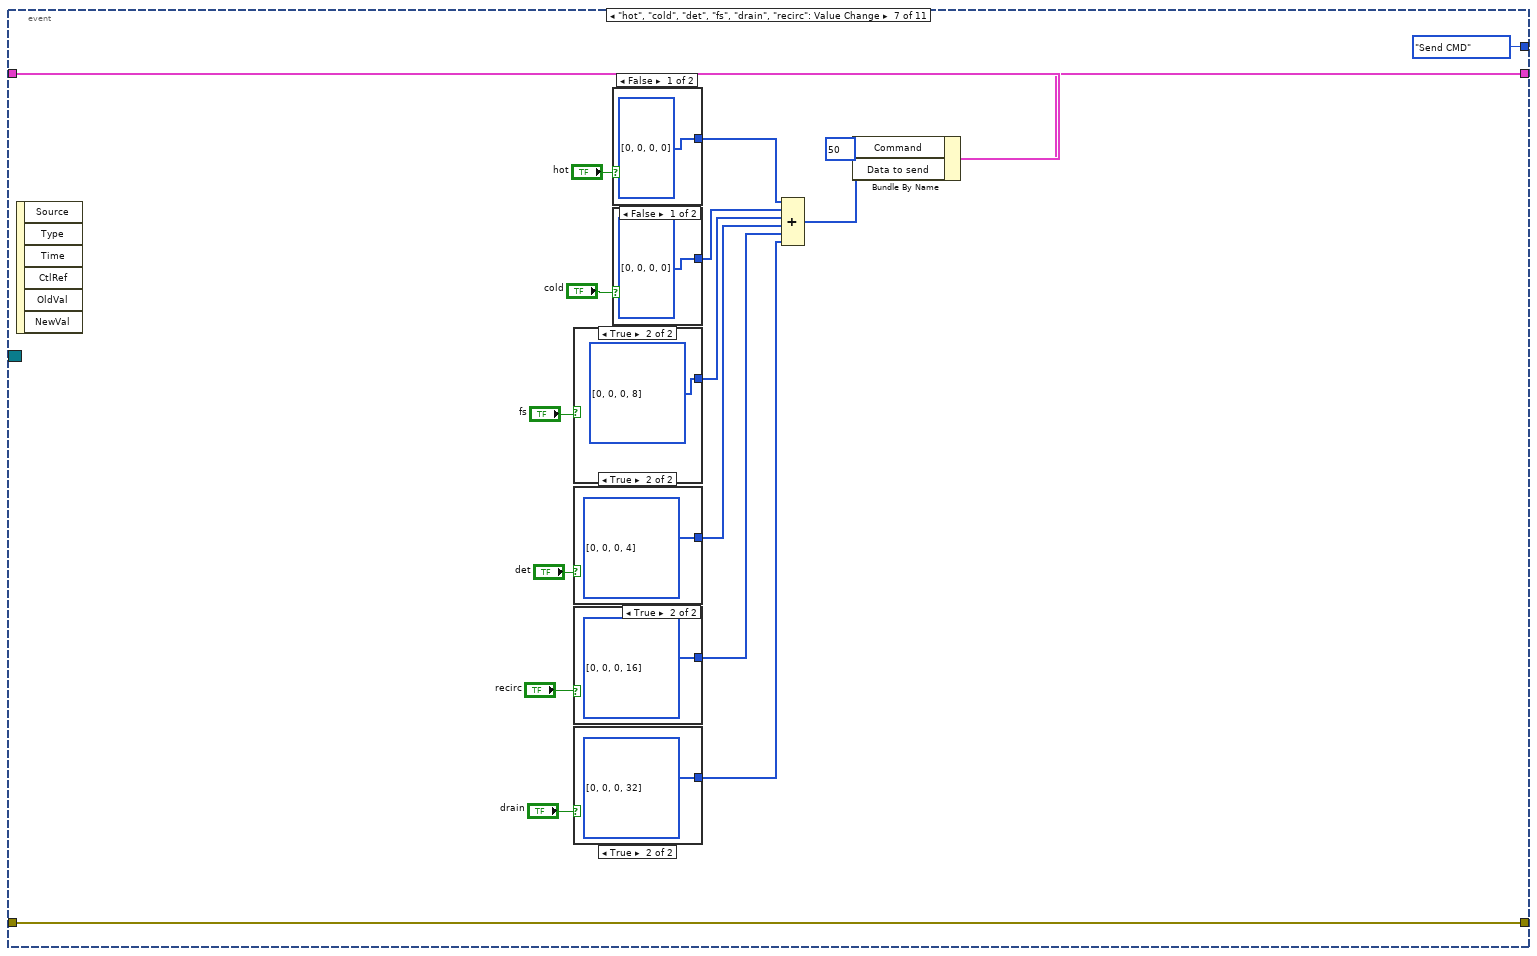
[diagram p19: hidden frame]
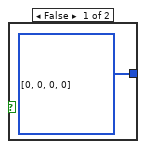
[diagram p20: hidden frame]
diagram:
  w5 = TRUE  # NufiDataRead
  n1 = flat-sequence {
    tunnel: ["Macro: Initialize\n"] -> w9
    frame #0 {
      w13 = FALSE ("Complete?")
      w12 = 0.0 ("Total Gallons")
      n2 = local write "Enter File Init State"(w13) -> ()
      n3 = local write "All Fields Complete"(w13) -> ()
      n4 = local write "Total Gallons Cold"(w12) -> ()
      n5 = local write "Total Gallons Hot"(w12) -> ()
      n6 = local write "Complete?"(w13) -> ()
      n7 = local write "Elapsed Time"(w12) -> ()
    }
  }
  n8 = Create User Event(user event datatype=w5) -> (user event=w4:refnum<user-event>)  [unwired: 1 in, 1 out]
  n9 = register-events(w4) -> (reference out=w3:refnum<event-registration>)  [unwired: 2 in, 1 out]
  n10 = call <vilib>:"Add State(s) to Queue__jki_lib_state_machine.vi"("State(s) in (\"\")"=w9) -> ("States Out"=w11:string)  [unwired: 14 in]
  n11 = while {
    shift-right: [w24] -> _
    shift-left: T8 {"GEA2 Message Ref"=refnum, "Board ID"="", "USB Connect"=refnum, "GEA Bus"=refnum, "Address"=0, "Source"=0, "Message Count"=0.0, "ReceivedData"=[], "Log?"=FALSE, "Partial Message String"="", "Full Message to Save"="", "Data to send"=[], "Command"=0, "selected path"=path "", "debugRef"=refnum, "dataRef"=refnum, "logData"={"IGBT Temp"=0, "Speed"=0, "Load Size"=0, "Temperature"=0, "Water Pressure"=0, "Detergent"=0, "Fabric Softener"=0, "Direction"="", "Det"=FALSE, "FS"=FALSE, "Recirc"=FALSE, "Drain"=FALSE, "Hot"=FALSE, "Cold"=FALSE, "LidClosed"=FALSE, "LidLocked"=FALSE}, "GraphData"=[]} ("Initialize") -> [w23]
    shift-right: [w17] -> w2
    shift-left: errorcluster {"status"=FALSE, "code"=0, "source"=""} ("error out") -> [w22]
    shift-right: [w18] -> _
    shift-left: States."Data" -> [w19]
    tunnel: w3 -> [w21]
    tunnel: w4 -> [w20]
    stop <- w15 stop-if-true
    n12 = case shown="\"Data\"" w19 {
      tunnel: w23 -> [w28 w39 w58 w61 w69 w244 w260 w356 w391 w415 w474 w522 w540 w573 w582 w598]
      tunnel: [w27 w34 w45 w62 w68 w254 w275 w363 w399 w432 w488 w524 w537 w574 w581 w586] -> w17
      tunnel: w22 -> [w27 w34 w53 w62 w67 w254 w275 w363 w399 w432 w488 w529 w541 w575 w581 w589]
      tunnel: [FALSE FALSE FALSE FALSE FALSE FALSE FALSE FALSE FALSE FALSE FALSE FALSE FALSE FALSE FALSE TRUE] -> w16
      tunnel: [w28 w40 w48 w61 w66 w243 w265 w354 w390 w414 w473 w521 w539 w572 w582 w598] -> w24
      tunnel: w21 -> [_ _ _ _ w65 _ _ _ _ _ _ _ _ _ _ _]
      tunnel: w20 -> [_ _ w52 _ _ _ _ _ _ _ _ _ _ _ _ _]
      tunnel: [States."Wait" States."GEA2" States."Wait" States."Wait" w63 w230 w268 States."Send CMD" States."Send CMD" States."Wait" States."Wait" States."Wait" w536 States."Update Graphs" States."Wait" States."Exit"] -> w18
      frame "-------- Initialize --------" {
      }
      frame "Data" {
        w33 = T11."Enabled" ("Disabled")
        w32 = T11."Disabled and Grayed Out" ("Disabled")
        n13 = property on="hot" class="Bool (strict)"("DisabledEnum"=w32) -> ()  [unwired: 2 in, 2 out]
        n14 = property on="StartLog" class="Bool"("DisabledEnum"=w32) -> ()  [unwired: 2 in, 2 out]
        n15 = property on="cold" class="Bool (strict)"("DisabledEnum"=w32) -> ()  [unwired: 2 in, 2 out]
        n16 = property on="fs" class="Bool (strict)"("DisabledEnum"=w32) -> ()  [unwired: 2 in, 2 out]
        n17 = property on="SaveGraph" class="Bool"("DisabledEnum"=w32) -> ()  [unwired: 2 in, 2 out]
        n18 = property on="det" class="Bool (strict)"("DisabledEnum"=w32) -> ()  [unwired: 2 in, 2 out]
        n19 = property on="StartLog" class="Bool"("DisabledEnum"=w32) -> ()  [unwired: 2 in, 2 out]
        n20 = property on="drain" class="Bool (strict)"("DisabledEnum"=w32) -> ()  [unwired: 2 in, 2 out]
        n21 = property on="recirc" class="Bool (strict)"("DisabledEnum"=w32) -> ()  [unwired: 2 in, 2 out]
        n22 = property on="Path" class="Bool"("DisabledEnum"=w33) -> ()  [unwired: 2 in, 2 out]
        n23 = property on="Path" class="Bool"("DisabledEnum"=w33) -> ()  [unwired: 2 in, 2 out]
        n24 = property on="EOL" class="Bool (strict)"("BoolText.Text"="Enter EOL" ("Boolean Text.Text")) -> ()  [unwired: 2 in, 2 out]
        n25 = property on="EOL" class="Bool (strict)"("Value"=FALSE ("EOL")) -> ()  [unwired: 2 in, 2 out]
        n26 = property on="Command:Data" class="Str"("Text.Text"="") -> ()  [unwired: 2 in, 2 out]
        n27 = Bundle By Name(cluster=w39, "Address"=u8 35, "Source"=u8 228) -> (w40:T8)
      }
      frame "GEA2" {
        # "Set up GEA2 USB connection"
        # "Send command to get UI version"
        n28 = Unbundle By Name(w58) -> ("Address"=w54:u8)
        n29 = call "GEA Initialize.vi"("NufiDataRead"=w52, "Address"=w54, "error in (no error)"=w53) -> (".NET Refnum out"=w47:refnum<k24>, "Running"=→"GEA2":bool, "Board ID"=w55:string, "error out"=w46:errorcluster)  [unwired: 13 in]
        "Board ID" <- w55
        n30 = Bundle By Name(cluster=w58, "GEA Bus"=w47, "Board ID"=w55) -> (w48:T8)
        n31 = Unbundle By Name(w48) -> ("Source"=w44:u8, "Address"=w43:u8)
        n32 = constructor class="GeaMessage"(error in=w46, "source"=w44, "destination"=w43, "command"=u8 1, "data"=u8[] []) -> (reference out=w49:refnum<k24>, error out=w50:errorcluster)  [unwired: 2 in, 5 out]
        n33 = invoke class="AbstractGeaBus" method="SendMessage"(reference=w47, error in=w50, "messageToSend"=w49) -> (error out=w45:errorcluster)  [unwired: 1 in, 3 out]
      }
      frame "---------- Core ----------" {
      }
      frame "Wait", Default {
        n34 = event shown="[10] \"Exit\", \"Stop\": Value Change" {
          selector: w65 -> [_ _ _ _ _ _ _ _ _ _ _]
          dyn-events: _ -> [_ _ _ _ _ _ _ _ _ _ _]
          timeout: _ -> [_ _ _ _ _ _ _ _ _ _ _]
          tunnel: w69 -> [w72 w112 w115 w133 w172 w177 w195 w211 w220 w226 w228]
          tunnel: [w75 w104 w117 w132 w155 w178 w196 w212 w215 w224 w229] -> w68
          tunnel: w67 -> [w75 w104 w117 w132 w161 w178 w196 w212 w215 w224 w229]
          tunnel: [w74 w112 w116 w133 w171 w176 w194 w211 w219 w225 w228] -> w66
          tunnel: [w73 States."Wait" States."Send CMD" States."Wait" States."Wait" States."Wait" States."Send CMD" States."Wait" States."Wait" States."Send CMD" States."Exit"] -> w63
          event User Event {
            n35 = event-data() -> ()  [unwired: 1 in, 5 out]
            n36 = global read "Nufi Global_ReceivedDataCluster.vi" "Nufi Data"() -> (w76:T12)
            n37 = Unbundle By Name(w76) -> ("ReceivedData"=w70:u8[], "Command"=w71:u8)
            n38 = case shown="1" w71 {
              tunnel: [States."Wait" States."Wait" States."Read MC Data" States."Read Incoder Position" States."Read Inv Data" States."Read Debug" States."Read LEDs"] -> w73
              tunnel: w70 -> [_ w98 _ _ _ _ _]
              frame 0, Default {
              }
              frame 1 {
                # "Parse UI version info coming back\nfrom command issued in GEA2 state"
                n39 = Reverse 1D Array(array=w98) -> (reversed array=w83:u8[])
                n40 = Index Array(array=w83, index #1=0 ("index")) -> (element #1=w96:u8, element #2=w95:u8)  [unwired: 1 in]
                n41 = Index Array(array=w83, index #1=4 ("index")) -> (element #1=w85:u8, element #2=w84:u8)  [unwired: 1 in]
                n42 = Index Array(array=w83, index=8) -> (element=w78:u8)
                n43 = Increment(x=w78) -> (x+1=w79:u8)
                n44 = Number To Decimal String(number=w96) -> (decimal integer string=w94:string)  [unwired: 1 in]
                n45 = Number To Decimal String(number=w95) -> (decimal integer string=w92:string)  [unwired: 1 in]
                n46 = Number To Decimal String(number=w85) -> (decimal integer string=w89:string)  [unwired: 1 in]
                n47 = Number To Decimal String(number=w84) -> (decimal integer string=w87:string)  [unwired: 1 in]
                n48 = Number To Decimal String(number=w79) -> (decimal integer string=→"Personality":string)  [unwired: 1 in]
                n49 = Concatenate Strings(w94, "." ("string"), w92) -> (→"UI Version":string)
                n50 = Concatenate Strings(w89, "." ("string"), w87) -> (→"Param. Ver.":string)
              }
              frame 65 {
              }
              frame 148 {
              }
              frame 96 {
              }
              frame 116 {
              }
              frame 159 {
              }
            }
            n51 = Bundle By Name(cluster=w72, "ReceivedData"=w70) -> (w74:T8)
          }
          event "SaveGraph": Value Change {
            (unwired) enum32{"File", "Clipboard"}."File" ("Target")
            (unwired) enum32{"BMP", "EPS", "EMF", "PICT"}."BMP" ("File Type")
            n52 = event-data() -> ()  [unwired: 1 in, 6 out]
            n53 = Unbundle By Name(w112) -> ("dataRef"=w110:refnum<file>)
            n54 = Get Date/Time In Seconds() -> (seconds since 1Jan1904=w108:timestamp)
            n55 = Refnum to Path(1:w110) -> (0:w111:path)
            n56 = Format Date/Time String(time format string (%c)="%b_%d__%H_%M_%S.bmp", seconds (now)=w108) -> (date/time string=w106:string)  [unwired: 1 in]
            n57 = Strip Path(path=w111) -> (stripped path=w105:path)  [unwired: 1 out]
            n58 = Build Path(base path=w105, name or relative path=w106) -> ()  [unwired: 1 out]
          }
          event "EOL": Value Change {
            n59 = event-data() -> ()  [unwired: 1 in, 6 out]
            n60 = case shown="False" "EOL" {
              tunnel: [w121 w130] -> w116
              tunnel: w115 -> [w122 w127]
              frame False {
                w118 = FALSE ("Value")
                w119 = T11."Disabled and Grayed Out" ("Disabled")
                n61 = property on="EOL" class="Bool (strict)"("BoolText.Text"="Enter EOL" ("Boolean Text.Text")) -> ()  [unwired: 2 in, 2 out]
                n62 = Bundle By Name(cluster=w122, "Command"=u8 144, "Data to send"=u8[] [0]) -> (w121:T8)
                n63 = property on="drain" class="Bool (strict)"("DisabledEnum"=w119) -> ()  [unwired: 2 in, 2 out]
                n64 = property on="cold" class="Bool (strict)"("DisabledEnum"=w119) -> ()  [unwired: 2 in, 2 out]
                n65 = property on="det" class="Bool (strict)"("DisabledEnum"=w119) -> ()  [unwired: 2 in, 2 out]
                n66 = property on="fs" class="Bool (strict)"("DisabledEnum"=w119) -> ()  [unwired: 2 in, 2 out]
                n67 = property on="hot" class="Bool (strict)"("DisabledEnum"=w119) -> ()  [unwired: 2 in, 2 out]
                n68 = property on="recirc" class="Bool (strict)"("DisabledEnum"=w119) -> ()  [unwired: 2 in, 2 out]
                n69 = property on="drain" class="Bool (strict)"("Value"=w118) -> ()  [unwired: 2 in, 2 out]
                n70 = property on="cold" class="Bool (strict)"("Value"=w118) -> ()  [unwired: 2 in, 2 out]
                n71 = property on="det" class="Bool (strict)"("Value"=w118) -> ()  [unwired: 2 in, 2 out]
                n72 = property on="fs" class="Bool (strict)"("Value"=w118) -> ()  [unwired: 2 in, 2 out]
                n73 = property on="hot" class="Bool (strict)"("Value"=w118) -> ()  [unwired: 2 in, 2 out]
                n74 = property on="Recirc" class="Bool (strict)"("Value"=w118) -> ()  [unwired: 2 in, 2 out]
              }
              frame True {
                w125 = T11."Enabled" ("Disabled")
                n75 = property on="EOL" class="Bool (strict)"("BoolText.Text"="Exit EOL" ("Boolean Text.Text")) -> ()  [unwired: 2 in, 2 out]
                n76 = Bundle By Name(cluster=w127, "Command"=u8 144, "Data to send"=u8[] [1]) -> (w130:T8)
                n77 = property on="drain" class="Bool (strict)"("DisabledEnum"=w125) -> ()  [unwired: 2 in, 2 out]
                n78 = property on="recirc" class="Bool (strict)"("DisabledEnum"=w125) -> ()  [unwired: 2 in, 2 out]
                n79 = property on="cold" class="Bool (strict)"("DisabledEnum"=w125) -> ()  [unwired: 2 in, 2 out]
                n80 = property on="hot" class="Bool (strict)"("DisabledEnum"=w125) -> ()  [unwired: 2 in, 2 out]
                n81 = property on="det" class="Bool (strict)"("DisabledEnum"=w125) -> ()  [unwired: 2 in, 2 out]
                n82 = property on="fs" class="Bool (strict)"("DisabledEnum"=w125) -> ()  [unwired: 2 in, 2 out]
              }
            }
          }
          event "Clear": Value Change {
            n83 = event-data() -> ()  [unwired: 1 in, 6 out]
            n84 = property on="Command:Data" class="Str"("Text.Text"="") -> ()  [unwired: 2 in, 2 out]
          }
          event "Path": Value Change {
            w137 = ","
            w151 = T11."Enabled" ("Disabled")
            w160 = T13."replace or create with confirmation" ("operation (0:open)")
            # "Header for data collection file"
            n85 = event-data() -> ()  [unwired: 1 in, 6 out]
            n86 = property on="Path" class="Bool"("DisabledEnum"=T11."Disabled and Grayed Out" ("Disabled")) -> ()  [unwired: 2 in, 2 out]
            n87 = property on="StartLog" class="Bool"("DisabledEnum"=w151) -> ()  [unwired: 2 in, 2 out]
            n88 = property on="SaveGraph" class="Bool"("DisabledEnum"=w151) -> ()  [unwired: 2 in, 2 out]
            n89 = call "File Dialog"("error in"=w161) -> ("selected path"=w166:path, "error out"=w162:errorcluster)  [unwired: 11 in, 2 out]
            n90 = Build Path(base path=w166, name or relative path="DebugLog.txt") -> (appended path=w165:path)
            n91 = Build Path(base path=w166, name or relative path="Data.csv") -> (appended path=w163:path)
            n92 = Open/Create/Replace File(file path (use dialog)=w165, error in=w162, operation (0:open)=w160) -> (refnum out=w156:refnum<file>, error out=w164:errorcluster)  [unwired: 3 in, 1 out]
            n93 = Concatenate Strings("Time" ("string"), w137, "Detergent Frequency" ("string"), w137, "Detergent Valve" ("string"), w137, "Fabric Softener Frequency" ("string"), w137, "Fabric Softener Valve" ("string"), w137, "Water Pressure" ("string"), w137, "Cold Valve" ("string"), w137, "Hot Valve" ("string"), w137, "Temperature" ("string"), w137, "Speed" ("string"), w137, "Load Size" ("string"), w137, "Direction" ("string"), w137, "Drain Pump" ("string"), w137, "Recirc Pump" ("string"), w137, "Lid Closed?" ("string"), w137, "Lid Locked?" ("string"), "\r") -> (w152:string)
            n94 = Open/Create/Replace File(file path (use dialog)=w163, error in=w164, operation (0:open)=w160) -> (refnum out=w158:refnum<file>, error out=w159:errorcluster)  [unwired: 3 in, 1 out]
            n95 = Write to Text File(file (use dialog)=w158, text=w152, error in=w159) -> (refnum out=w157:refnum<file>, error out=w155:errorcluster)  [unwired: 1 in, 1 out]
            n96 = Bundle By Name(cluster=w172, "debugRef"=w156, "dataRef"=w157) -> (w171:T8)
          }
          event "StartLog": Value Change {
            n97 = event-data() -> ()  [unwired: 1 in, 6 out]
            n98 = property on="StartLog" class="Bool"("DisabledEnum"=T11."Disabled and Grayed Out" ("Disabled")) -> ()  [unwired: 2 in, 2 out]
            n99 = Bundle By Name(cluster=w177, "Log?"=TRUE) -> (w176:T8)
          }
          event "hot", "cold", "det", "fs", "drain", "recirc": Value Change {
            n100 = event-data() -> ()  [unwired: 1 in, 6 out]
            n101 = case shown="True" "fs" {
              tunnel: [u8[] [0, 0, 0, 0] ("Data to send") u8[] [0, 0, 0, 8] ("Data to send")] -> w188
              frame False {
              }
              frame True {
              }
            }
            n102 = case shown="True" "det" {
              tunnel: [u8[] [0, 0, 0, 0] ("Data to send") u8[] [0, 0, 0, 4] ("Data to send")] -> w184
              frame False {
              }
              frame True {
              }
            }
            n103 = case shown="True" "recirc" {
              tunnel: [u8[] [0, 0, 0, 0] ("Data to send") u8[] [0, 0, 0, 16] ("Data to send")] -> w183
              frame False {
              }
              frame True {
              }
            }
            n104 = case shown="True" "drain" {
              tunnel: [u8[] [0, 0, 0, 0] ("Data to send") u8[] [0, 0, 0, 32] ("Data to send")] -> w182
              frame False {
              }
              frame True {
              }
            }
            n105 = case shown="False" "hot" {
              tunnel: [u8[] [0, 0, 0, 0] ("Data to send") u8[] [0, 0, 1, 0] ("Data to send")] -> w186
              frame False {
              }
              frame True {
              }
            }
            n106 = case shown="False" "cold" {
              tunnel: [u8[] [0, 0, 0, 0] ("Data to send") u8[] [0, 0, 2, 0] ("Data to send")] -> w187
              frame False {
              }
              frame True {
              }
            }
            n107 = Compound Arithmetic op=ADD(w186, w187, w188, w184, w183, w182) -> (w189:u8[])
            n108 = Bundle By Name(cluster=w195, "Command"=u8 50, "Data to send"=w189) -> (w194:T8)
          }
          event "Viper/Hawk": Value Change {
            n109 = event-data() -> ()  [unwired: 1 in, 6 out]
            n110 = case shown="1" "Viper/Hawk" {
              frame 0, Default {
                w213 = TRUE ("Visible")
                # "Viper"
                n111 = property on="Fabric Softener" class="DigNum (strict)"("Visible"=w213) -> ()  [unwired: 2 in, 2 out]
                n112 = property on="Detergent" class="DigNum (strict)"("Visible"=w213) -> ()  [unwired: 2 in, 2 out]
                n113 = property on="Det" class="Bool (strict)"("Visible"=w213) -> ()  [unwired: 2 in, 2 out]
                n114 = property on="FS" class="Bool (strict)"("Visible"=w213) -> ()  [unwired: 2 in, 2 out]
                n115 = property on="det" class="Bool (strict)"("Visible"=w213) -> ()  [unwired: 2 in, 2 out]
                n116 = property on="fs" class="Bool (strict)"("Visible"=w213) -> ()  [unwired: 2 in, 2 out]
              }
              frame 1 {
                w214 = FALSE ("Visible")
                # "Hawk"
                n117 = property on="Fabric Softener" class="DigNum (strict)"("Visible"=w214) -> ()  [unwired: 2 in, 2 out]
                n118 = property on="Detergent" class="DigNum (strict)"("Visible"=w214) -> ()  [unwired: 2 in, 2 out]
                n119 = property on="Det" class="Bool (strict)"("Visible"=w214) -> ()  [unwired: 2 in, 2 out]
                n120 = property on="det" class="Bool (strict)"("Visible"=w214) -> ()  [unwired: 2 in, 2 out]
                n121 = property on="fs" class="Bool (strict)"("Visible"=w214) -> ()  [unwired: 2 in, 2 out]
                n122 = property on="FS" class="Bool (strict)"("Visible"=w214) -> ()  [unwired: 2 in, 2 out]
              }
            }
          }
          event "Address", "Source": Value Change {
            n123 = event-data() -> ()  [unwired: 1 in, 6 out]
            n124 = Bundle By Name(cluster=w220, "Address"="Address", "Source"="Source") -> (w219:T8)
          }
          event "Send": Value Change {
            n125 = event-data() -> ()  [unwired: 1 in, 6 out]
            n126 = Bundle By Name(cluster=w226, "Command"="Command", "Data to send"="Data") -> (w225:T8)
          }
          event "Exit", "Stop": Value Change {
            n127 = event-data() -> ()  [unwired: 1 in, 6 out]
          }
        }
      }
      frame "Read Debug" {
        w234 = 5000 ("length (rest)")
        w247 = ""  # Msg Delimiter
        n128 = Unbundle By Name(w244) -> ("Log?"=w231:bool, "Partial Message String"=w246:string, "ReceivedData"=w253:u8[])
        n129 = Reverse 1D Array(array=w253) -> (reversed array=w232:u8[])
        n130 = Byte Array To String(unsigned byte array=w232) -> (string=w245:string)
        n131 = call "Nufi Dryer Debug Message Buff.vi"("New String"=w245, "Partial Message String"=w246) -> ("Partial Message FWD"=w241:string, "Full Message to Save"=w242:string)  [unwired: 7 in, 1 out]
        n132 = Concatenate Strings("Command:Data", w247, w245) -> (w239:string)
        n133 = String Length(string=w239) -> (length=w238:i32)
        n134 = Subtract(x=w238, y=w234) -> (x-y=w237:i32)
        n135 = In Range and Coerce(upper limit=w234, x=w237, lower limit=0) -> (coerced(x)=w236:i32)  [unwired: 1 out]
        n136 = String Subset(string=w239, offset (0)=w236, length (rest)=w234) -> (substring=w240:string)
        n137 = Search and Replace String(input string=w240, search string="\n") -> (number of replacements=w250:i32)  [unwired: 6 in, 3 out]
        n138 = Bundle By Name(cluster=w244, "Full Message to Save"=w242, "Partial Message String"=w241) -> (w243:T8)
        n139 = case shown="True" w231 {
          tunnel: [States."Wait" States."Log Debug"] -> w230
          frame False {
          }
          frame True {
          }
        }
        n140 = Subtract(x=w250, y=10) -> (x-y=w252:i32)
        n141 = property on="Command:Data" class="Str"("Text.Scroll Position"=w252) -> ()  [unwired: 2 in, 2 out]
        n142 = property on="Command:Data" class="Str"("Text.Text"=w240) -> ()  [unwired: 2 in, 2 out]
      }
      frame "Read MC Data" {
        w259 = ""
        n143 = Unbundle By Name(w260) -> ("ReceivedData"=w274:u8[])
        n144 = Reverse 1D Array(array=w274) -> (reversed array=w264:u8[])
        n145 = for {
          tunnel: w264 -> [w294] mode=indexing
          shift-right: [w289] -> w271
          shift-left: w259 -> [w290]
          shift-right: [w288] -> w270
          shift-left: w259 -> [w286]
          shift-right: [w284] -> w272
          shift-left: w259 -> [w283]
          shift-right: [w282] -> w269
          shift-left: w259 -> [w281]
          shift-right: [w278] -> w263
          shift-left: w260 -> [w279]
          i -> [w292]
          n146 = Increment(x=w292) -> (x+1=w293:i32)
          n147 = case shown="5" w293 {
            tunnel: w294 -> [_ w298 w305 w313 w317 w321 w327 w331 w334 w339 w343 w347 w351]
            tunnel: [w296 _ _ _ w316 w320 _ _ _ _ _ _ _] -> w291
            tunnel: [w296 _ _ _ _ _ _ w330 w333 _ _ _ _] -> w287
            tunnel: [w296 _ _ _ _ _ _ _ _ w338 w342 _ _] -> w285
            tunnel: [w296 _ _ _ _ _ _ _ _ _ _ w346 w350] -> w280
            tunnel: w279 -> [w295 w299 w303 w311 w315 w319 w325 w329 w335 w337 w341 w345 w349]
            tunnel: [w295 w297 w302 w310 w315 w319 w322 w329 w335 w337 w341 w345 w349] -> w278
            frame 0, Default {
              w296 = ""
            }
            frame 1 {
              n148 = Bundle By Name(cluster=w299, "logData.Temperature"=w298) -> (w297:T8)
              "Temperature" <- w298
            }
            frame 4 {
              n149 = Number To Boolean Array(number=w305) -> (Boolean array=w304:bool[])
              n150 = Index Array(array=w304) -> (element #1=w301:bool, element #2=w300:bool)  [unwired: 2 in]
              "Hot" <- w301
              "Cold" <- w300
              n151 = Bundle By Name(cluster=w303, "logData.Hot"=w301, "logData.Cold"=w300) -> (w302:T8)
              n152 = Boolean To (0,1)(Boolean=w300) -> ()  [unwired: 1 out]
              n153 = Boolean To (0,1)(Boolean=w301) -> ()  [unwired: 1 out]
            }
            frame 5 {
              n154 = Number To Boolean Array(number=w313) -> (Boolean array=w312:bool[])
              n155 = Index Array(array=w312) -> (element #3=w309:bool, element #4=w308:bool, element #5=w307:bool, element #6=w306:bool)  [unwired: 6 in, 2 out]
              "Det" <- w309
              "FS" <- w308
              "Recirc" <- w307
              "Drain" <- w306
              n156 = Bundle By Name(cluster=w311, "logData.Det"=w309, "logData.FS"=w308, "logData.Recirc"=w307, "logData.Drain"=w306) -> (w310:T8)
            }
            frame 6 {
              # "water pressure"
              n157 = Number To Hexadecimal String(1:i16 2 ("width (-)"), 2:w317) -> (0:w316:string)
            }
            frame 7 {
              # "water pressure"
              n158 = Number To Hexadecimal String(1:i16 2 ("width (-)"), 2:w321) -> (0:w320:string)
            }
            frame 10 {
              n159 = Number To Boolean Array(number=w327) -> (Boolean array=w326:bool[])
              n160 = Index Array(array=w326) -> (element #1=w324:bool, element #2=w323:bool)  [unwired: 2 in]
              "Lid Closed?" <- w324
              "Lid Locked?" <- w323
              n161 = Bundle By Name(cluster=w325, "logData.LidClosed"=w324, "logData.LidLocked"=w323) -> (w322:T8)
            }
            frame 15 {
              # "detergent"
              n162 = Number To Hexadecimal String(1:i16 2 ("width (-)"), 2:w331) -> (0:w330:string)
            }
            frame 16 {
              # "detergent"
              n163 = Number To Hexadecimal String(1:i16 2 ("width (-)"), 2:w334) -> (0:w333:string)
            }
            frame 17 {
              # "fs"
              n164 = Number To Hexadecimal String(1:i16 2 ("width (-)"), 2:w339) -> (0:w338:string)
            }
            frame 18 {
              # "fs"
              n165 = Number To Hexadecimal String(1:i16 2 ("width (-)"), 2:w343) -> (0:w342:string)
            }
            frame 25 {
              # "hall sensor"
              n166 = Number To Hexadecimal String(1:i16 2 ("width (-)"), 2:w347) -> (0:w346:string)
            }
            frame 26 {
              # "hall sensor"
              n167 = Number To Hexadecimal String(1:i16 2 ("width (-)"), 2:w351) -> (0:w350:string)
            }
          }
          n168 = Concatenate Strings(w281, w280) -> (w282:string)
          n169 = Concatenate Strings(w286, w287) -> (w288:string)
          n170 = Concatenate Strings(w283, w285) -> (w284:string)
          n171 = Concatenate Strings(w290, w291) -> (w289:string)
        }
        n172 = Hexadecimal String To Number(string=w270) -> (number=w266:u32)  [unwired: 2 in, 1 out]
        "Detergent" <- w266
        n173 = Hexadecimal String To Number(string=w271) -> (number=w267:u32)  [unwired: 2 in, 1 out]
        "Water Pressure" <- w267
        n174 = Hexadecimal String To Number(string=w269) -> (number=w258:u32)  [unwired: 2 in, 1 out]
        "Speed" <- w258
        n175 = Hexadecimal String To Number(string=w272) -> (number=w261:u32)  [unwired: 2 in, 1 out]
        "Fabric Softener" <- w261
        n176 = Unbundle By Name(w260) -> ("Log?"=w262:bool)
        n177 = Bundle By Name(cluster=w263, "logData.Fabric Softener"=w261, "logData.Detergent"=w266, "logData.Water Pressure"=w267, "logData.Speed"=w258, "Command"=u8 148) -> (w265:T8)
        n178 = case shown="False" w262 {
          tunnel: [States."Send CMD" States."Log Data"] -> w268
          frame False {
          }
          frame True {
          }
        }
      }
      frame "Read Inv Data" {
        n179 = Unbundle By Name(w356) -> ("ReceivedData"=w362:u8[])
        n180 = Reverse 1D Array(array=w362) -> (reversed array=w360:u8[])
        n181 = for {
          tunnel: w360 -> [w371] mode=indexing
          shift-right: [w368] -> w358
          shift-left: "" -> [w367]
          shift-right: [w365] -> w355
          shift-left: w356 -> [w364]
          i -> [w369]
          n182 = Increment(x=w369) -> (x+1=w370:i32)
          n183 = case shown="0, Default" w370 {
            tunnel: w371 -> [_ w377 w382 w384 w386]
            tunnel: ["" _ w381 w385 _] -> w366
            tunnel: w364 -> [w372 w376 w380 w383 w388]
            tunnel: [w372 w375 w380 w383 w387] -> w365
            frame 0, Default {
            }
            frame 1 {
              n184 = case shown="0, Default" w377 {
                tunnel: ["cw" ("String") "ccw" ("String")] -> w374
                frame 0, Default {
                }
                frame 1 {
                }
              }
              "Direction" <- w374
              n185 = Bundle By Name(cluster=w376, "logData.Direction"=w374) -> (w375:T8)
            }
            frame 4 {
              # "load size"
              n186 = Number To Hexadecimal String(2:w382) -> (0:w381:string)  [unwired: 1 in]
            }
            frame 5 {
              # "load size"
              n187 = Number To Hexadecimal String(2:w384) -> (0:w385:string)  [unwired: 1 in]
            }
            frame 10 {
              n188 = Bundle By Name(cluster=w388, "logData.IGBT Temp"=w386) -> (w387:T8)
            }
          }
          n189 = Concatenate Strings(w367, w366) -> (w368:string)
        }
        n190 = Hexadecimal String To Number(string=w358) -> (number=w353:u32)  [unwired: 2 in, 1 out]
        "Load Size" <- w353
        n191 = Bundle By Name(cluster=w355, "logData.Load Size"=w353, "Command"=u8 148) -> (w354:T8)
      }
      frame "Read Incoder Position" {
        n192 = Unbundle By Name(w391) -> ("ReceivedData"=w398:u8[])
        n193 = Reverse 1D Array(array=w398) -> (reversed array=w395:u8[])
        n194 = Index Array(array=w395, index=0) -> (element=w393:u8)
        n195 = case shown="15" w393 {
          tunnel: ["Normal" "Towels/Sheets" "Sanitize" "Bulky Items" "Quick Rinse" "Drain & Spin" "Basket Clean" "Speedwash" "Delicates" "Jeans" "Heavy Duty" "Dark Colors" "Whites"] -> w392
          frame 0, Default {
          }
          frame 1 {
          }
          frame 2 {
          }
          frame 3 {
          }
          frame 4 {
          }
          frame 5 {
          }
          frame 6 {
          }
          frame 10 {
          }
          frame 11 {
          }
          frame 12 {
          }
          frame 13 {
          }
          frame 14 {
          }
          frame 15 {
          }
        }
        "Incoder Position" <- w392
        n196 = Bundle By Name(cluster=w391, "Command"=u8 148) -> (w390:T8)
      }
      frame "Read LEDs" {
        # "Pre-Soak Setting"
        # "Spin Setting"
        # "Temp Settings"
        # "Soil Settings"
        n197 = Unbundle By Name(w415) -> ("ReceivedData"=w431:u8[])
        n198 = Reverse 1D Array(array=w431) -> (reversed array=w428:u8[])
        n199 = Index Array(array=w428, index=21) -> (element=w416:u8)
        n200 = Index Array(array=w428, index=11) -> (element=w422:u8)
        n201 = Index Array(array=w428, index=9) -> (element=w421:u8)
        n202 = Index Array(array=w428, index=8) -> (element=w423:u8)
        n203 = case shown="0, Default" w423 {
          tunnel: ["Extra Light" "Light" "Normal" "Heavy" "Extra Heavy"] -> w417
          frame 0, Default {
          }
          frame 1 {
          }
          frame 2 {
          }
          frame 3 {
          }
          frame 4 {
          }
        }
        "Soil Setting" <- w417
        n204 = case shown="0, Default" w421 {
          tunnel: ["Tap Cold" "Cold" "Cool" "Colors" "Warm" "Hot"] -> w418
          frame 0, Default {
          }
          frame 1 {
          }
          frame 2 {
          }
          frame 3 {
          }
          frame 4 {
          }
          frame 5 {
          }
        }
        "Temperature Setting" <- w418
        n205 = case shown="0, Default" w416 {
          tunnel: ["Off" "30 Minutes" "1 Hour" "1:30 Hours" "2 Hours"] -> w420
          frame 0, Default {
          }
          frame 1 {
          }
          frame 2 {
          }
          frame 3 {
          }
          frame 4 {
          }
        }
        "Pre Soak" <- w420
        n206 = case shown="0, Default" w422 {
          tunnel: ["No Spin" "Low" "Medium" "High" "Extra High"] -> w419
          frame 0, Default {
          }
          frame 1 {
          }
          frame 2 {
          }
          frame 3 {
          }
          frame 4 {
          }
        }
        "Spin Setting" <- w419
        n207 = Bundle By Name(cluster=w415, "Command"=u8 148) -> (w414:T8)
      }
      frame "Update Graphs" {
        n208 = Unbundle By Name(w474) -> ("logData"=w477:T9, "GraphData"=w475:T9[])
        n209 = Index Array(array=w475) -> (element=w478:T9)  [unwired: 1 in]
        n210 = Build Array(w477) -> (w476:T9[])
        n211 = Equal?(x=w478, y=T9 {"IGBT Temp"=0, "Speed"=0, "Load Size"=0, "Temperature"=0, "Water Pressure"=0, "Detergent"=0, "Fabric Softener"=0, "Direction"="", "Det"=FALSE, "FS"=FALSE, "Recirc"=FALSE, "Drain"=FALSE, "Hot"=FALSE, "Cold"=FALSE, "LidClosed"=FALSE, "LidLocked"=FALSE} ("logData")) -> (x = y?=w485:T14)
        n212 = Cluster To Array(cluster=w485) -> (array=w484:bool[])
        n213 = And Array Elements(Boolean array=w484) -> (logical AND=w483:bool)
        n214 = case shown="True" w483 {
          tunnel: w475 -> [w514 w516]
          tunnel: [w514 w515] -> w479
          frame False {
          }
          frame True {
            n215 = Delete From Array(array=w516, index=0) -> (array with subset deleted=w515:T9[])  [unwired: 1 in, 1 out]
          }
        }
        n216 = Array Size(array=w479) -> (size(s)=w482:i32)
        n217 = Greater Or Equal?(x=w482, y=241) -> (x >= y?=w480:bool)
        n218 = case shown="False" w480 {
          tunnel: w479 -> [w505 w510]
          tunnel: [w507 w511] -> w455
          tunnel: w476 -> [w506 w512]
          frame False {
            n219 = Insert Into Array(array=w505, index=0, new element=w506) -> (w507:T9[])
          }
          frame True {
            n220 = Delete From Array(array=w510, index=240) -> (array with subset deleted=w508:T9[])  [unwired: 1 in, 1 out]
            n221 = Insert Into Array(array=w508, index=0, new element=w512) -> (w511:T9[])
          }
        }
        n222 = for {
          tunnel: w455 -> [w503] mode=indexing
          tunnel: [w502] -> w456 mode=indexing
          tunnel: [w501] -> w457 mode=indexing
          tunnel: [w500] -> w458 mode=indexing
          tunnel: [w499] -> w459 mode=indexing
          tunnel: [w497] -> w460 mode=indexing
          tunnel: [w495] -> w467 mode=indexing
          tunnel: [w494] -> w468 mode=indexing
          tunnel: [w491] -> w469 mode=indexing
          tunnel: [w490] -> w470 mode=indexing
          n223 = Unbundle By Name(w503) -> ("Water Pressure"=w502:u32, "Speed"=w501:u32, "Temperature"=w500:u8, "Cold"=w498:bool, "Hot"=w496:bool, "Detergent"=w495:u32, "Fabric Softener"=w494:u32, "Det"=w493:bool, "FS"=w492:bool)
          n224 = Boolean To (0,1)(Boolean=w492) -> (0, 1=w490:i16)
          n225 = Boolean To (0,1)(Boolean=w493) -> (0, 1=w491:i16)
          n226 = Boolean To (0,1)(Boolean=w496) -> (0, 1=w497:i16)
          n227 = Boolean To (0,1)(Boolean=w498) -> (0, 1=w499:i16)
        }
        n228 = Reverse 1D Array(array=w456) -> (reversed array=w454:u32[])
        n229 = Reverse 1D Array(array=w457) -> (reversed array=w461:u32[])
        n230 = Reverse 1D Array(array=w458) -> (reversed array=w462:u8[])
        n231 = Reverse 1D Array(array=w459) -> (reversed array=w463:i16[])
        n232 = Reverse 1D Array(array=w460) -> (reversed array=w464:i16[])
        n233 = Reverse 1D Array(array=w467) -> (reversed array=w465:u32[])
        n234 = Reverse 1D Array(array=w468) -> (reversed array=w466:u32[])
        n235 = Reverse 1D Array(array=w469) -> (reversed array=w471:i16[])
        n236 = Reverse 1D Array(array=w470) -> (reversed array=w472:i16[])
        n237 = Bundle(w454, w461, w462, w463, w464, w465, w466, w471, w472) -> ()  [unwired: 1 in, 1 out]
        n238 = Bundle By Name(cluster=w474, "GraphData"=w455) -> (w473:T8)
      }
      frame "Send CMD" {
        n239 = Unbundle By Name(w522) -> ("GEA Bus"=w530:refnum<k24>, "Source"=w518:u8, "Address"=w519:u8, "Command"=w527:u8, "Data to send"=w526:u8[])
        n240 = constructor class="GeaMessage"(error in=w529, "source"=w518, "destination"=w519, "command"=w527, "data"=w526) -> (reference out=w531:refnum<k24>, error out=w532:errorcluster)  [unwired: 2 in, 5 out]
        n241 = invoke class="AbstractGeaBus" method="SendMessage"(reference=w530, error in=w532, "messageToSend"=w531) -> (reference out=w520:refnum<k24>, error out=w525:errorcluster)  [unwired: 1 in, 2 out]
        n242 = Bundle By Name(cluster=w522, "GEA Bus"=w520) -> (w521:T8)
        n243 = flat-sequence {
          tunnel: w525 -> [w533]
          tunnel: [w533] -> w524
          frame #0 {
            n244 = Wait (ms)(milliseconds to wait=u32 100) -> ()  [unwired: 1 out]
          }
        }
      }
      frame "Log Debug" {
        w551 = -1 ("offset past match")
        # "if no eol delimiter, add one."
        n245 = Unbundle By Name(w540) -> ("logData.Recirc"=w535:bool, "debugRef"=w542:refnum<file>, "Full Message to Save"=w544:string)
        n246 = Get Date/Time String(date format (0)=enum16{"short", "long", "abbreviated"}."short", want seconds? (F)=TRUE) -> (time string=w564:string)  [unwired: 1 in, 1 out]
        n247 = Concatenate Strings(w564, " " ("string"), w544) -> (w545:string)
        n248 = Match Pattern(string=w545, regular expression="\r\n") -> (offset past match=w554:i32)  [unwired: 1 in, 3 out]
        n249 = Match Pattern(string=w545, regular expression="\n") -> (offset past match=w553:i32)  [unwired: 1 in, 3 out]
        n250 = Match Pattern(string=w545, regular expression="\r") -> (offset past match=w552:i32)  [unwired: 1 in, 3 out]
        n251 = Not Equal?(x=w554, y=w551) -> (x != y?=w550:bool)
        n252 = Not Equal?(x=w553, y=w551) -> (x != y?=w549:bool)
        n253 = Not Equal?(x=w552, y=w551) -> (x != y?=w548:bool)
        n254 = Compound Arithmetic op=AND(w550, w549, w548) -> (w547:bool)
        n255 = case shown="False" w547 {
          tunnel: [w567 w568] -> w546
          tunnel: w545 -> [w567 w570]
          frame False {
          }
          frame True {
            n256 = Concatenate Strings(w570, "\r\n") -> (w568:string)
          }
        }
        n257 = Set File Position(refnum=w542, from (0:start)=enum16{"start", "end", "current"}."end", error in=w541) -> (refnum out=w559:refnum<file>, error out=w560:errorcluster)  [unwired: 1 in]
        n258 = Write to Text File(file (use dialog)=w559, text=w546, error in=w560) -> (refnum out=w538:refnum<file>, error out=w537:errorcluster)  [unwired: 1 in, 1 out]
        n259 = Bundle By Name(cluster=w540, "debugRef"=w538) -> (w539:T8)
        n260 = case shown="True" w535 {
          tunnel: [States."Wait" States."Test"] -> w536
          frame False {
          }
          frame True {
          }
        }
      }
      frame "Log Data" {
        n261 = Unbundle By Name(w573) -> ("dataRef"=w576:refnum<file>, "logData"=w578:T9)
        n262 = call "formatLogData.vi"("input cluster"=w578) -> ("concatenated string"=w577:string)  [unwired: 18 in]
        n263 = Write to Text File(file (use dialog)=w576, text=w577, error in=w575) -> (refnum out=w571:refnum<file>, error out=w574:errorcluster)  [unwired: 1 in, 1 out]
        n264 = Bundle By Name(cluster=w573, "dataRef"=w571) -> (w572:T8)
      }
      frame "Test" {
      }
      frame "Exit" {
        w596 = FALSE ("Exit")
        # "Stop GEA Bus"
        n265 = property on="Exit" class="Bool (strict)"("Value"=w596) -> ()  [unwired: 2 in, 2 out]
        n266 = property on="GEA2" class="Bool (strict)"("Value"=w596) -> ()  [unwired: 2 in, 2 out]
        n267 = Unbundle By Name(w598) -> ("dataRef"=w585:refnum<file>, "debugRef"=w597:refnum<file>, "GEA Bus"=w591:refnum<k24>, "GEA2 Message Ref"=w590:refnum<k24>)
        n268 = Close Reference(reference=w590, error in (no error)=w589) -> (error out=w593:errorcluster)
        n269 = invoke class="AbstractGeaBus" method="Stop"(reference=w591, error in=w593) -> (reference out=w595:refnum<k24>, error out=w594:errorcluster)  [unwired: 1 in, 1 out]
        n270 = Close Reference(reference=w595, error in (no error)=w594) -> (error out=w592:errorcluster)
        n271 = Close File(refnum=w597, error in=w592) -> (error out=w587:errorcluster)  [unwired: 1 out]
        n272 = Close File(refnum=w585, error in=w587) -> (error out=w586:errorcluster)  [unwired: 1 out]
      }
    }
    n273 = Or(x=w16, y=w17) -> (x .or. y?=w15:bool)
  }
  "error out" <- w2
  n274 = while "Main Control Loop" {
    shift-right: [w610] -> _
    shift-left: _ -> [w609]
    shift-right: [w613] -> _
    shift-left: _ -> [w608]
    shift-right: [w612] -> _
    shift-left: w11 -> [w614]
    shift-right: [w606] -> _
    shift-left: dbl[][] [] -> [w607]
    shift-right: [w600] -> _
    shift-left: string[][] [] -> [w601]
    stop <- w611 stop-if-true
    n275 = call <vilib>:"Parse State Queue__jki_lib_state_machine.vi"("State Queue"=w614, "Error In (no error)"=w608) -> ("Remaining States"=w616:string, "Current State"=w617:string, "Arguments"=w615:string)  [unwired: 11 in]
    "Current State" <- w617
    n276 = local read "Elapsed Time"() -> (w604:dbl)
    n277 = call "E-Time.vi"() -> ("Elapsed Time (sec)"=w602:dbl)  [unwired: 9 in, 2 out]
    n278 = call "RLT Timeout Calc.vi"("Complete time"=w602, "Gather Data Period"=1000, "Start Time"=w604) -> ("coerced(x)"=w603:i32)  [unwired: 8 in]
    n279 = case shown="\"File Initial\"" w617 {
      selector: w617 -> [_ _ w713 _ _ _ _ _ _ _ _ _ _ _ _ _ _ _ _ _ _ _ _ _ _ _ _ _ _ _ _]
      tunnel: w616 -> [w626 w710 w717 w738 w746 w753 w759 w805 w836 w845 w880 w888 w897 w911 w926 w935 w941 w947 w955 w968 w996 w1003 w1015 w1021 w1029 w1043 w1060 w1102 w1162 w1209 w1247]
      tunnel: w615 -> [_ _ _ _ _ _ _ _ _ _ _ _ _ _ _ _ _ _ w950 w962 _ _ _ _ _ _ _ _ _ _ _]
      tunnel: w609 -> [w624 w707 w715 w729 w743 w751 w756 w764 w829 w841 _ w885 w895 w908 w919 w930 w938 w942 w953 w964 w993 w1000 w1012 w1018 w1025 w1034 w1051 w1093 w1155 w1175 w1238]
      tunnel: [w623 w708 w719 w735 errorcluster {"status"=FALSE, "code"=0, "source"=""} ("error out") w750 w757 w763 w834 w843 w877 w886 w891 w905 w920 w931 w939 w945 w951 w965 w994 w1001 w1013 w1019 w1023 w1041 w1057 w1098 w1157 w1206 w1245] -> w613
      tunnel: w608 -> [w622 w708 w718 w735 w742 w750 w757 w763 w834 w843 w877 w886 w892 w905 w921 w932 w939 w945 w952 w966 w994 w1001 w1013 w1019 w1023 w1041 w1058 w1100 w1158 w1206 w1245]
      tunnel: [w625 w709 w716 w737 w745 w752 w758 w777 w835 w844 w879 w887 w896 w910 w925 w934 w940 w946 w954 w967 w995 w1002 w1014 w1020 w1024 w1042 w1059 w1101 w1161 w1208 w1246] -> w612
      tunnel: [_ _ _ _ _ TRUE _ _ _ _ _ _ _ _ _ _ _ _ _ _ _ _ _ _ _ _ _ _ _ _ _] -> w611
      tunnel: [w621 w707 w715 w736 w743 w751 w756 w764 w830 w841 w878 w885 w895 w907 w918 w930 w938 w942 w953 w964 w993 w1000 w1012 w1018 w1027 w1036 w1055 w1095 w1154 w1175 w1237] -> w610
      tunnel: w607 -> [w620 w706 w712 w726 w740 w748 w755 w804 w833 w842 w869 w883 w890 w909 w924 w929 w937 w944 w949 w961 w992 w998 w1005 w1017 w1028 w1039 w1048 w1091 w1148 w1207 w1243]
      tunnel: [w620 w706 w712 w726 w740 w748 w755 w804 w833 w842 w869 w883 w890 w909 w924 w929 w937 w944 w949 w961 w992 w998 w1005 w1017 w1028 w1039 w1048 w1091 w1148 w1207 w1242] -> w606
      tunnel: w603 -> [w619 _ _ _ _ _ _ _ _ _ _ _ _ _ _ _ _ _ _ _ _ _ _ _ _ _ _ _ _ _ _]
      tunnel: w601 -> [w618 w705 w711 w725 w739 w747 w754 w803 w832 w837 w861 w882 w889 w906 w913 w928 w936 w943 w948 w960 w991 w997 w1004 w1016 w1022 w1030 w1047 w1077 w1145 w1179 w1240]
      tunnel: [w618 w705 w711 w725 w739 w747 w754 w803 w832 w837 w861 w882 w889 w906 w913 w928 w936 w943 w948 w960 w991 w997 w1004 w1016 w1022 w1030 w1047 w1077 w1145 w1178 w1235] -> w600
      frame "", "Idle" {
        n280 = event shown="[1] \"File Setup OK\": Value Change" {
          selector: _ -> [_ _ _ _ _ _ _ _]
          dyn-events: _ -> [_ _ _ _ _ _ _ _]
          timeout: w619 -> [_ _ _ _ _ _ _ _]
          tunnel: w626 -> [w636 w641 w646 w654 w658 w663 w669 w704]
          tunnel: [w635 w640 w645 w653 w659 w664 w668 w704] -> w625
          tunnel: w624 -> [w628 w643 w647 w651 w657 w662 w667 w700]
          tunnel: [w634 w642 w648 w652 w655 w660 w665 w703] -> w623
          tunnel: w622 -> [w634 w642 w648 w652 w655 w660 w665 w703]
          tunnel: [w628 w643 w647 w651 w657 w662 w667 w699] -> w621
          event Timeout {
            n281 = event-data() -> ()  [unwired: 1 in, 1 out]
            n282 = Unbundle By Name(w628) -> ("Complete DOE Cap"=w627:bool)
            n283 = local read "Enter File Init State"() -> (w632:bool)
            n284 = local read "All Fields Complete"() -> (w631:bool)
            n285 = local read "Complete?"() -> (w629:bool)
            n286 = Compound Arithmetic op=AND(w632, w631, w629, w627) -> (w630:bool)
            n287 = case shown="False" w630 {
              tunnel: ["" "Init Laurel Meter\nInit WattHours\nInit Time\nInitialize Array\nUI Update\nGather Analog Data\nGather Flow Rates\nGet Power Data\nCheck Newfi\nShow Data"] -> w633
              frame False {
              }
              frame True {
              }
            }
            n288 = call <vilib>:"Add State(s) to Queue__jki_lib_state_machine.vi"("State(s) in Front (\"\")"=w633, "State(s) in (\"\")"=w636) -> ("States Out"=w635:string)  [unwired: 13 in]
          }
          event "File Setup OK": Value Change {
            n289 = event-data() -> ()  [unwired: 1 in, 6 out]
            n290 = call <vilib>:"Add State(s) to Queue__jki_lib_state_machine.vi"("State(s) in Front (\"\")"="File Initial", "State(s) in (\"\")"=w641) -> ("States Out"=w640:string)  [unwired: 13 in]
          }
          event "Complete DOE Cap": Value Change {
            n291 = event-data() -> ()  [unwired: 1 in, 6 out]
            n292 = call <vilib>:"Add State(s) to Queue__jki_lib_state_machine.vi"("State(s) in Front (\"\")"="DOE Capacity" ("State(s) in Front (\"\")"), "State(s) in (\"\")"=w646) -> ("States Out"=w645:string)  [unwired: 13 in]
          }
          event Panel Close? {
            n293 = event-data() -> ()  [unwired: 1 in, 1 out]
            n294 = call <vilib>:"Add State(s) to Queue__jki_lib_state_machine.vi"("State(s) in Front (\"\")"="Macro: Exit", "State(s) in (\"\")"=w654) -> ("States Out"=w653:string)  [unwired: 13 in]
            n295 = event-data("Discard?"=TRUE) -> ()  [unwired: 1 in, 1 out]
          }
          event "Start": Value Change {
            n296 = event-data() -> ()  [unwired: 1 in, 6 out]
            n297 = call <vilib>:"Add State(s) to Queue__jki_lib_state_machine.vi"("State(s) in Front (\"\")"="Macro: Initialize", "State(s) in (\"\")"=w658) -> ("States Out"=w659:string)  [unwired: 13 in]
          }
          event "Reset All": Value Change {
            n298 = event-data() -> ()  [unwired: 1 in, 6 out]
            n299 = call <vilib>:"Add State(s) to Queue__jki_lib_state_machine.vi"("State(s) in Front (\"\")"="Macro: Initialize", "State(s) in (\"\")"=w663) -> ("States Out"=w664:string)  [unwired: 13 in]
          }
          event "Stop": Value Change {
            n300 = event-data() -> ()  [unwired: 1 in, 6 out]
            n301 = call <vilib>:"Add State(s) to Queue__jki_lib_state_machine.vi"("State(s) in Front (\"\")"="Macro: Exit", "State(s) in (\"\")"=w669) -> ("States Out"=w668:string)  [unwired: 13 in]
          }
          event "Viper": Value Change {
            n302 = event-data() -> ()  [unwired: 1 in, 6 out]
            n303 = Unbundle By Name(w700) -> ("DOE Capacity Path"=w702:path)
            n304 = call-poly <vilib>:"Read From Spreadsheet File.vi"("delimiter (\\t)"="," ("delimiter (\\t)"), "file path (dialog if empty)"=w702) -> ("all rows"=w697:string[][])  [unwired: 5 in, 4 out]
            n305 = call "Extract Capacity Rows.vi"("Row"=0 ("disabled index (col)"), "all rows"=w697) -> ("Capacity Data"=w693:T18)  [unwired: 9 in]
            n306 = call "Extract Capacity Rows.vi"("Row"=1, "all rows"=w697) -> ("Capacity Data"=w687:T18)  [unwired: 9 in]
            n307 = call "Extract Capacity Rows.vi"("Row"=2, "all rows"=w697) -> ("Capacity Data"=w681:T18)  [unwired: 9 in]
            n308 = call "Extract Capacity Rows.vi"("Row"=3, "all rows"=w697) -> ("Capacity Data"=w675:T18)  [unwired: 9 in]
            n309 = Unbundle By Name(w681) -> ("Measured Temp"=w680:dbl, "Weight of Water"=w679:dbl, "Lab Number"=w678:string, "Serial Number"=w677:string, "Model Number"=w676:string)
            n310 = Unbundle By Name(w687) -> ("Measured Temp"=w686:dbl, "Weight of Water"=w685:dbl, "Lab Number"=w684:string, "Serial Number"=w683:string, "Model Number"=w682:string)
            n311 = property on="Measured Temp (Deg F )1" class="DigNum (strict)"("Value"=w686) -> ()  [unwired: 2 in, 2 out]
            n312 = property on="Weight of Water (lbs)1" class="DigNum (strict)"("Value"=w685) -> ()  [unwired: 2 in, 2 out]
            n313 = property on="Lab Number1" class="Str"("Value"=w684) -> ()  [unwired: 2 in, 2 out]
            n314 = property on="Serial Number1" class="Str"("Value"=w683) -> ()  [unwired: 2 in, 2 out]
            n315 = property on="Model Number1" class="Str"("Value"=w682) -> ()  [unwired: 2 in, 2 out]
            n316 = property on="Measured Temp (Deg F)2" class="DigNum (strict)"("Value"=w680) -> ()  [unwired: 2 in, 2 out]
            n317 = property on="Weight of Water (lbs)2" class="DigNum (strict)"("Value"=w679) -> ()  [unwired: 2 in, 2 out]
            n318 = property on="Lab Number2" class="Str"("Value"=w678) -> ()  [unwired: 2 in, 2 out]
            n319 = property on="Serial Number2" class="Str"("Value"=w677) -> ()  [unwired: 2 in, 2 out]
            n320 = property on="Model Number2" class="Str"("Value"=w676) -> ()  [unwired: 2 in, 2 out]
            n321 = Unbundle By Name(w675) -> ("Measured Temp"=w670:dbl, "Weight of Water"=w671:dbl, "Lab Number"=w672:string, "Serial Number"=w673:string, "Model Number"=w674:string)
            n322 = Unbundle By Name(w693) -> ("Measured Temp"=w692:dbl, "Weight of Water"=w691:dbl, "Lab Number"=w690:string, "Serial Number"=w689:string, "Model Number"=w688:string)
            n323 = Bundle By Name(cluster=w700, "Washer 1"=w693, "Washer 2"=w687, "Washer 3"=w681, "Washer 4"=w675) -> (w699:T19)
            n324 = property on="Measured Temp (Deg F)3" class="DigNum (strict)"("Value"=w670) -> ()  [unwired: 2 in, 2 out]
            n325 = property on="Weight of Water (lbs)3" class="DigNum (strict)"("Value"=w671) -> ()  [unwired: 2 in, 2 out]
            n326 = property on="Lab Number3" class="Str"("Value"=w672) -> ()  [unwired: 2 in, 2 out]
            n327 = property on="Serial Number3" class="Str"("Value"=w673) -> ()  [unwired: 2 in, 2 out]
            n328 = property on="Model Number3" class="Str"("Value"=w674) -> ()  [unwired: 2 in, 2 out]
            n329 = property on="Measured Temp" class="DigNum (strict)"("Value"=w692) -> ()  [unwired: 2 in, 2 out]
            n330 = property on="Water Weight" class="DigNum (strict)"("Value"=w691) -> ()  [unwired: 2 in, 2 out]
            n331 = property on="Lab Number" class="Str"("Value"=w690) -> ()  [unwired: 2 in, 2 out]
            n332 = property on="Serial Number" class="Str"("Value"=w689) -> ()  [unwired: 2 in, 2 out]
            n333 = property on="Model Number" class="Str"("Value"=w688) -> ()  [unwired: 2 in, 2 out]
          }
        }
      }
      frame "---------- Core ----------" {
        n334 = call <vilib>:"Add State(s) to Queue__jki_lib_state_machine.vi"("State(s) in (\"\")"=w710) -> ("States Out"=w709:string)  [unwired: 14 in]
      }
      frame Default {
        w722 = 42 items=["No error", "Argument error", "Memory is full", "Out of zone", "End of file", "File already open", "Generic file I/O error", "File not found", "File permission error", "Disk is full", "Duplicate path", "Too many files open", "System feature not enabled", "Resource file not found", "Cannot add resource", "Resource not found", "Image not found", "Image memory error", "Pen does not exist", "Config type invalid", "Config token not found", "Config parse error", "Config memory error", "Bad external code format", "Bad external code offset", "External code not present", "Null window", "Destroy window error", "Null menu", "Print aborted", "Bad print record", "Print driver error", "Windows error during printing", "Memory error during printing", "Print dialog error", "Generic print error", "Invalid device refnum", "Device not found", "Device parameter error", "Device unit error", "Cannot open device", "Device call aborted", "Generic error", "Cancelled by user", "Object ID too low", "Object ID too high", "Object not in heap", "Unknown heap", "Unknown object (invalid DefProc)", "Unknown object (DefProc not in table)", "Message out of range", "Invalid (null) method", "Unknown message", "Manager call not supported", "Bad address", "Network operation in progress", "Network operation timed out", "Connection is busy", "Network attribute not supported", "Network error", "Address in use", "System out of memory", "Connection aborted", "Connection refused", "Not connected", "Already connected", "Connection closed", "Initialization error (interapplication manager)", "Bad occurrence", "Wait on unbound occurrence handler", "Occurrence queue overflow", "Datalog type conflict", "Unused", "Unrecognized type (interapplication manager)", "Memory corrupt", "Failed to make temporary DLL", "Old CIN version", "Drag socket not found", "Failed to load drop-object", "Failed to register OLE object", "Failed to release OLE object", "Format specifier type mismatch", "Unknown format specifier", "Too few format specifiers", "Too many format specifiers", "Scan failed", "Newer CIN version", "Error converting to variant", "Runtime menu error", "Password tampered", "Variant attribute not found", "Incompatible variant data type", "Event data is not available", "Event Store is not present", "Occurrence is not found", "Event Queue is not created", "Event info is not available", "Refnum passed is NULL", "Error retrieving Class GUID", "Error retrieving CoClass GUID", "Error retrieving TypeLib GUID.", "Bad built application magic bytes.", "Specific driver is different from the specific driver associated with the Logical Name.", "There is no session opened to the class driver.", "Max Error", "MAX - Error with config objects", "MAX - Error loading configuration", "MAX - Group not supported"]
        # "Current State"
        # "Handle mistyped state name (developer tool)"
        n335 = call <vilib>:"Add State(s) to Queue__jki_lib_state_machine.vi"("State(s) in (\"\")"=w717) -> ("States Out"=w716:string)  [unwired: 14 in]
        n336 = Format Into String(format string="Software Exception: Unhandled State \"%s\"." ("message"), error in=w718, w713) -> (resulting string=w721:string, error out=w720:errorcluster)  [unwired: 1 in]
        n337 = call <vilib>:"Error Cluster From Error Code.vi"("show call chain? (False)"=TRUE, "error in (no error)"=w720, "error message (\"\")"=w721, "error code (0)"=w722) -> ("error out"=w719:errorcluster)  [unwired: 5 in]
      }
      frame "Initialize Core Data" {
        # "Switch The Tab"
        # "originally closed?"
        # "exe?"
        # "If panel starts closed or is an EXE, then close it when we exit"
        n338 = call <vilib>:"Add State(s) to Queue__jki_lib_state_machine.vi"("State(s) in (\"\")"=w738) -> ("States Out"=w737:string)  [unwired: 14 in]
        n339 = property class="App"() -> ("App.Kind"=w733:T15)  [unwired: 2 in, 2 out]
        n340 = property class="VI"() -> ("Front Panel.Open"=w734:bool)  [unwired: 2 in, 2 out]
        n341 = control-ref of="Current VI Reference"() -> (w727:refnum<vi>)
        n342 = Equal?(x=w733, y=T15."Run Time System" ("Application:Kind")) -> (x = y?=w730:bool)
        n343 = Not(x=w734) -> (.not. x?=w731:bool)
        n344 = Or(x=w731, y=w730) -> (x .or. y?=w728:bool)
        n345 = Bundle By Name(cluster=w729, "Core.Current VI Reference"=w727, "Core.Close Panel on Exit?"=w728) -> (w736:T19)
        n346 = local write "Tab Control 3"(T2."DOE Capacity Testing" ("Tab Control 3")) -> ()
      }
      frame "Error Handler" {
        n347 = call <vilib>:"General Error Handler.vi"("error in (no error)"=w742) -> ()  [unwired: 10 in, 5 out]
        n348 = call <vilib>:"Add State(s) to Queue__jki_lib_state_machine.vi"("State(s) in Front (\"\")"="/* Post Error States", "State(s) in (\"\")"=w746) -> ("States Out"=w745:string)  [unwired: 13 in]
      }
      frame "Exit" {
        n349 = call <vilib>:"Add State(s) to Queue__jki_lib_state_machine.vi"("State(s) in (\"\")"=w753) -> ("States Out"=w752:string)  [unwired: 14 in]
      }
      frame "---------- Data ----------" {
        n350 = call <vilib>:"Add State(s) to Queue__jki_lib_state_machine.vi"("State(s) in (\"\")"=w759) -> ("States Out"=w758:string)  [unwired: 14 in]
      }
      frame "File Initial" {
        w768 = ""
        w771 = "_"
        n351 = call <vilib>:"Add State(s) to Queue__jki_lib_state_machine.vi"("State(s) in (\"\")"=w805) -> ("States Out"=w778:string)  [unwired: 14 in]
        n352 = Unbundle By Name(w764) -> ("All Models Excel Sheet"=w760:path, "Network Model Location"=w762:path)
        n353 = Get Date/Time In Seconds() -> (seconds since 1Jan1904=w802:timestamp)
        "Test Date:" <- w802
        n354 = case shown="0, Default" "Station ID:" {
          tunnel: ["No Station Selected" "Station 1" "Station 2" "Station 3" "Station 4" "Station 5" "Station 6" "Station 7" "Station 8"] -> w789
          frame 0, Default {
          }
          frame 1 {
          }
          frame 2 {
          }
          frame 3 {
          }
          frame 4 {
          }
          frame 5 {
          }
          frame 6 {
          }
          frame 7 {
          }
          frame 8 {
          }
        }
        n355 = Get Date/Time String(seconds (now)=w802) -> (date string=w798:string)  [unwired: 2 in, 1 out]
        n356 = call "Model Number and Folder Setup.vi"("Network Model Location"=w762, "All Models Excel Sheet"=w760) -> ("Model Data"=→"Model Information":string[][])  [unwired: 9 in]
        n357 = for {
          N: 2 -> [_]
          shift-right: [w814] -> w796
          shift-left: w798 -> [w817]
          n358 = Search and Replace String(input string=w817, search string="/", replace string="-" ("replace string (\"\")")) -> (result string=w814:string)  [unwired: 5 in, 3 out]
        }
        n359 = Number To Fractional String(number="Capacity (cu.ft):", precision (6)=i16 3) -> (F-format string=w770:string)  [unwired: 2 in]
        n360 = Number To Fractional String(number="Initial Cloth Weight", precision (6)=i16 3) -> (F-format string=w769:string)  [unwired: 2 in]
        n361 = Equal?(x="Model Number:", y=w768) -> (x = y?=w787:bool)
        n362 = Equal?(x="Serial Number:", y=w768) -> (x = y?=w786:bool)
        n363 = Equal?(x="Engineering ID:", y=w768) -> (x = y?=w785:bool)
        n364 = Equal?(x="Lab ID:", y=w768) -> (x = y?=w784:bool)
        n365 = Equal?(x="Technician:", y=w768) -> (x = y?=w783:bool)
        n366 = Equal?(x=w770, y="0.000") -> (x = y?=w782:bool)
        n367 = Equal?(x=w789, y="No Station Selected") -> (x = y?=w781:bool)
        n368 = Equal?(x=w769, y="0.000") -> (x = y?=w767:bool)
        n369 = Concatenate Strings("Model Number:", w771, "Serial Number:", w771, "Engineering ID:", w771, "Lab ID:", w771, "Technician:", w771, w789, w771, w770, w771, w769, w771, w771, w796, ".xlsx" ("string")) -> (w779:string)
        n370 = Compound Arithmetic op=OR(w787, w786, w785, w784, w783, w782, w781, w767) -> (w780:bool)
        n371 = case shown="True" w780 {
          tunnel: w779 -> [w809 _]
          tunnel: [w808 w811] -> w775
          frame False {
            w808 = TRUE
            n372 = String To Path(string=w809) -> (path=→"File Path":path)
            "All Fields Complete" <- w808
          }
          frame True {
            w811 = FALSE ("All Fields Complete")
            n373 = local write "All Fields Complete"(w811) -> ()
            n374 = One Button Dialog(message="Required Fields:\nModel Number\nSerial Number\nEngineering ID\nLab ID\nTechnician\nStation ID\nCapacity (cu.ft)\nInitial Cloth Weigth", button name ("OK")="OK") -> ()  [unwired: 1 out]
          }
        }
        n375 = case shown="True" w775 {
          tunnel: ["" w807] -> w776
          frame False {
          }
          frame True {
            w807 = "Initialize Core Data\nUI: Initialize\nUI: Front Panel State >> Open\n"  # Initialize Core Data UI: Initialize UI: Front Panel State >> Open
          }
        }
        n376 = call <vilib>:"Add State(s) to Queue__jki_lib_state_machine.vi"("State(s) in Front (\"\")"=w776, "State(s) in (\"\")"=w778) -> ("States Out"=w777:string)  [unwired: 13 in]
        "Enter File Init State" <- TRUE ("Enter File Init State")
      }
      frame "Equipment" {
        n377 = Unbundle By Name(w829) -> ("Calibration File Path"=w827:path)
        n378 = call <vilib>:"Add State(s) to Queue__jki_lib_state_machine.vi"("State(s) in (\"\")"=w836) -> ("States Out"=w835:string)  [unwired: 14 in]
        n379 = call "Calibration.vi"("Show Front Panel"=TRUE, "file path (dialog if empty)"=w827) -> ("OutputData"=w828:string[][])  [unwired: 8 in, 1 out]
        n380 = Bundle By Name(cluster=w829, "Calibration"=w828) -> (w830:T19)
      }
      frame "Init WattHours" {
        n381 = call <vilib>:"Add State(s) to Queue__jki_lib_state_machine.vi"("State(s) in (\"\")"=w845) -> ("States Out"=w844:string)  [unwired: 14 in]
        n382 = Unbundle By Name(w841) -> ("Aplus IP Address"=w840:string, "Remote Port"=w839:i32)
        n383 = call "APLUS Camille Bauer Driver.vi"("Reset WattHours"=TRUE, "Remote Port"=w839, "Remote IP Address"=w840) -> ()  [unwired: 7 in, 2 out]
      }
      frame "Data: Initialize" {
        (unwired) T20 {"Calibration File Path"=path "", "DOE Capacity Path"=path "", "All Models Excel Sheet"=path "", "Network Model Location"=path ""} ("cluster")
        w859 = string[][] []  # Calibration
        w871 = dbl[] []  # Total Array
        w872 = 0.0  # Watt Hours
        w873 = T21 {"Voltage"=0.0, "Current"=0.0, "Frequency"=0.0, "Power"=0.0, "Power Factor"=0.0}  # Power
        w876 = T22 {"Current VI Reference"=refnum, "Close Panel on Exit?"=FALSE}  # Core
        n384 = local read "Test Date:"() -> (→"Test Date:DOE Cap":timestamp)
        n385 = local read "Technician:"() -> (→"Technician:DOE Cap":string)
        n386 = call <vilib>:"Add State(s) to Queue__jki_lib_state_machine.vi"("State(s) in (\"\")"=w880) -> ("States Out"=w879:string)  [unwired: 14 in]
        n387 = Bundle("Calibration File Path"="Calibration File Path", "DOE Capacity Path"="DOE Capacity Path", "All Models Excel Sheet"="All Models Excel Sheet", "Network Model Location"="Network Model Location") -> (w847:T20)  [unwired: 1 in]
        n388 = Bundle("Core"=w876, "Remote Port"="Remote Port", "Aplus IP Address"="Aplus IP Address", "Power"=w873, "Watt Hours"=w872, "Total Array"=w871, "VISA Laurel Meter"="VISA Laurel Meter", "FrontPanel Meters 2"="FrontPanel Meters 2", "Total Gallons Cold"="Total Gallons Cold", "Total Gallons Hot"="Total Gallons Hot", "2015?"="2015?", "Off Mode Watts"="Off Mode Watts", "Standby Mode Watts"="Standby Mode Watts", "Low Power Switch"="Low Power Switch", "First Time Through"="First Time Through", "Calibration"=w859, "Washer 1"="Washer 1", "Washer 2"="Washer 2", "Washer 3"="Washer 3", "Washer 4"="Washer 4", w847, "Complete DOE Cap"="Complete DOE Cap") -> (w878:T19)  [unwired: 1 in]
        n389 = local write "Tab Control 3"(T2."File Setup" ("Tab Control 3")) -> ()
      }
      frame "Init Time" {
        n390 = call "E-Time.vi"("Reset"=TRUE) -> ("Elapsed Time (sec)"=→"Start Time (sec)":dbl)  [unwired: 8 in, 2 out]
        n391 = call <vilib>:"Add State(s) to Queue__jki_lib_state_machine.vi"("State(s) in (\"\")"=w888) -> ("States Out"=w887:string)  [unwired: 14 in]
      }
      frame "Init Laurel Meter" {
        n392 = Unbundle By Name(w895) -> ("VISA Laurel Meter"=w894:refnum<visa-resource-name>)
        n393 = call "Laurel Meter Serial.vi"("error in (no error)"=w892, "VISA resource name"=w894, "Send Command"=T16."Cold Reset") -> ("error out"=w891:errorcluster)  [unwired: 7 in, 1 out]
        n394 = call <vilib>:"Add State(s) to Queue__jki_lib_state_machine.vi"("State(s) in (\"\")"=w897) -> ("States Out"=w896:string)  [unwired: 14 in]
      }
      frame "DOE Capacity" {
        n395 = Unbundle By Name(w908) -> ("Washer 1"=w904:T6, "Washer 2"=w903:T5, "Washer 3"=w902:T4, "Washer 4"=w901:T3)
        n396 = local write "Tab Control 3"(T2."Front Panel" ("Tab Control 3")) -> ()
        n397 = Bundle By Name(cluster=w908, "Washer 1"=w904, "Washer 2"=w903, "Washer 3"=w902, "Washer 4"=w901, "Complete DOE Cap"=TRUE) -> (w907:T19)
        n398 = call <vilib>:"Add State(s) to Queue__jki_lib_state_machine.vi"("State(s) in Front (\"\")"="Off-Standby Mode\nEquipment" ("State(s) in Front (\"\")"), "State(s) in (\"\")"=w911) -> ("States Out"=w910:string)  [unwired: 13 in]
      }
      frame "Off-Standby Mode" {
        n399 = Unbundle By Name(w919) -> ("Aplus IP Address"=w923:string, "Remote Port"=w922:i32)
        n400 = call "Off Mode Standby Mode Power Measure SM.vi"("Aplus IP Address"=w923, "Remote Port"=w922, "Error In"=w921) -> ("Complete?"=→"Complete?":bool, "Off Mode Watts"=w917:dbl, "2015 Output"=w916:bool, "Standby Watts"=w915:dbl, "Low Power Switch"=w914:bool, "Error Out"=w920:errorcluster)  [unwired: 7 in]
        n401 = call <vilib>:"Add State(s) to Queue__jki_lib_state_machine.vi"("State(s) in (\"\")"=w926) -> ("States Out"=w925:string)  [unwired: 14 in]
        n402 = Bundle By Name(cluster=w919, "Off Mode Watts"=w917, "2015?"=w916, "Standby Mode Watts"=w915, "Low Power Switch"=w914) -> (w918:T19)
      }
      frame "Data: Cleanup" {
        n403 = Unbundle By Name(w930) -> ("Core.Current VI Reference"=w933:refnum<vi>)
        n404 = Close Reference(reference=w933, error in (no error)=w932) -> (error out=w931:errorcluster)
        n405 = call "Counter.vi"("Reset"=TRUE) -> ()  [unwired: 10 in, 1 out]
        n406 = call <vilib>:"Add State(s) to Queue__jki_lib_state_machine.vi"("State(s) in (\"\")"=w935) -> ("States Out"=w934:string)  [unwired: 14 in]
      }
      frame "---------- UI ----------" {
        n407 = call <vilib>:"Add State(s) to Queue__jki_lib_state_machine.vi"("State(s) in (\"\")"=w941) -> ("States Out"=w940:string)  [unwired: 14 in]
      }
      frame "UI: Initialize" {
        n408 = call <vilib>:"Add State(s) to Queue__jki_lib_state_machine.vi"("State(s) in (\"\")"=w947) -> ("States Out"=w946:string)  [unwired: 14 in]
      }
      frame "UI: Cursor Set" {
        n409 = case shown="\"Idle\", Default" w950 {
          tunnel: w952 -> [w957 w959]
          tunnel: [w956 w958] -> w951
          frame "Idle", Default {
            n410 = call <vilib>:"Unset Busy.vi"("error in (no error)"=w957) -> ("error out"=w956:errorcluster)  [unwired: 10 in]
          }
          frame "Busy" {
            n411 = call <vilib>:"Set Busy.vi"("error in (no error)"=w959) -> ("error out"=w958:errorcluster)  [unwired: 9 in, 1 out]
          }
        }
        n412 = call <vilib>:"Add State(s) to Queue__jki_lib_state_machine.vi"("State(s) in (\"\")"=w955) -> ("States Out"=w954:string)  [unwired: 14 in]
      }
      frame "UI: Front Panel State" {
        n413 = Unbundle By Name(w964) -> ("Core.Current VI Reference"=w963:refnum<vi>)
        n414 = case shown="\"Open\", Default" w962 {
          tunnel: w966 -> [w972 w985]
          tunnel: [w974 w986] -> w965
          tunnel: w963 -> [w973 w983]
          frame "Open", Default {
            n415 = property class="VI"(reference=w973, error in=w972) -> (reference out=w970:refnum<vi>, error out=w971:errorcluster, "Front Panel.Open"=w969:bool)
            n416 = case shown="True" w969 {
              tunnel: [w977 w980] -> w974
              tunnel: w971 -> [w976 w980]
              tunnel: w970 -> [w975 _]
              frame False {
                n417 = invoke class="VI" method="FP.Open"(reference=w975, error in=w976, "Activate"=TRUE, "State"=T17."Standard") -> (error out=w977:errorcluster)  [unwired: 1 in, 4 out]
              }
              frame True {
              }
            }
          }
          frame "Close" {
            n418 = property class="VI"(reference=w983, error in=w985) -> (reference out=w982:refnum<vi>, error out=w984:errorcluster, "Front Panel.Open"=w981:bool)
            n419 = case shown="True" w981 {
              tunnel: [w987 w990] -> w986
              tunnel: w984 -> [w987 w989]
              tunnel: w982 -> [_ w988]
              frame False {
              }
              frame True {
                n420 = invoke class="VI" method="FP.Close"(reference=w988, error in=w989) -> (error out=w990:errorcluster)  [unwired: 1 in, 2 out]
              }
            }
          }
        }
        n421 = call <vilib>:"Add State(s) to Queue__jki_lib_state_machine.vi"("State(s) in (\"\")"=w968) -> ("States Out"=w967:string)  [unwired: 14 in]
      }
      frame "---------- Macro ----------" {
        n422 = call <vilib>:"Add State(s) to Queue__jki_lib_state_machine.vi"("State(s) in (\"\")"=w996) -> ("States Out"=w995:string)  [unwired: 14 in]
      }
      frame "Macro: Initialize" {
        n423 = call <vilib>:"Add State(s) to Queue__jki_lib_state_machine.vi"("State(s) in Front (\"\")"="Data: Initialize\n", "State(s) in (\"\")"=w1003) -> ("States Out"=w1002:string)  [unwired: 13 in]
      }
      frame "Macro: Exit" {
        n424 = Unbundle By Name(w1012) -> ("Core.Close Panel on Exit?"=w1011:bool)
        n425 = Select(t="UI: Front Panel State >> Close", s=w1011, f="") -> (s? t:f=w1008:string)
        n426 = call <vilib>:"Add State(s) to Queue__jki_lib_state_machine.vi"("State(s) in (\"\")"=w1008, "State(s) at Back (\"\")"="Data: Cleanup\nExit") -> ("States Out"=w1006:string)  [unwired: 13 in]
        n427 = call <vilib>:"Add State(s) to Queue__jki_lib_state_machine.vi"("State(s) in Front (\"\")"=w1006, "State(s) in (\"\")"=w1015) -> ("States Out"=w1014:string)  [unwired: 13 in]
      }
      frame "---------- New Category ----------" {
        n428 = call <vilib>:"Add State(s) to Queue__jki_lib_state_machine.vi"("State(s) in (\"\")"=w1021) -> ("States Out"=w1020:string)  [unwired: 14 in]
      }
      frame "Initialize Array" {
        n429 = call <vilib>:"Add State(s) to Queue__jki_lib_state_machine.vi"("State(s) in (\"\")"=w1029) -> ("States Out"=w1024:string)  [unwired: 14 in]
        n430 = Bundle By Name(cluster=w1025, "Total Array"=dbl[] []) -> (w1027:T19)
      }
      frame "UI Update" {
        n431 = local read "Elapsed Time"() -> (w1033:dbl)
        n432 = Unbundle By Name(w1034) -> ("Total Array"=w1038:dbl[])
        n433 = call "E-Time.vi"() -> ("Elapsed Time (sec)"=w1032:dbl)  [unwired: 9 in, 2 out]
        "Elapsed Time (sec)" <- w1032
        n434 = local read "Start Time (sec)"() -> (w1040:dbl)
        n435 = Subtract(x=w1032, y=w1033) -> (x-y=→"Loop Time":dbl)
        n436 = Subtract(x=w1032, y=w1040) -> (x-y=w1037:dbl)
        "Elapsed Time" <- w1037
        n437 = Build Array (concatenate)(w1038, w1037) -> (w1035:dbl[])
        n438 = call <vilib>:"Add State(s) to Queue__jki_lib_state_machine.vi"("State(s) in (\"\")"=w1043) -> ("States Out"=w1042:string)  [unwired: 14 in]
        n439 = Bundle By Name(cluster=w1034, "Total Array"=w1035) -> (w1036:T19)
      }
      frame "Gather Analog Data" {
        n440 = Unbundle By Name(w1051) -> ("Total Array"=w1050:dbl[])
        n441 = call "Advantech.vi"("error in (no error)"=w1058) -> ("error out"=w1057:errorcluster, "Advantech"=w1056:T23)  [unwired: 9 in]
        n442 = Unbundle By Name(w1056) -> ("Cold Water Pressure"=w1052:dbl, "Hot Water Pressure"=w1054:dbl, "Cold Water Temp"=w1046:dbl, "Hot Water Temp"=w1045:dbl, "Ambient Temp"=w1044:dbl, "Room Humidity"=w1053:dbl)
        n443 = Build Array (concatenate)(w1050, w1052, w1054, w1046, w1045, w1044, w1053) -> (w1049:dbl[])
        n444 = Bundle By Name(cluster=w1051, "Total Array"=w1049, "FrontPanel Meters 2.Cold Water\nPressure"=w1052, "FrontPanel Meters 2.Hot Water\nPressure"=w1054, "FrontPanel Meters 2.Cold Water\nTemperature"=w1046, "FrontPanel Meters 2.Hot Water\nTemperature"=w1045) -> (w1055:T19)
        n445 = call <vilib>:"Add State(s) to Queue__jki_lib_state_machine.vi"("State(s) in (\"\")"=w1060) -> ("States Out"=w1059:string)  [unwired: 14 in]
      }
      frame "Gather Flow Rates" {
        n446 = Delete From Array(array=w1077, index (col)=18 ("disabled index (col)")) -> (deleted portion=w1075:string[])  [unwired: 2 in, 1 out]
        n447 = call <vilib>:"Add State(s) to Queue__jki_lib_state_machine.vi"("State(s) in (\"\")"=w1102) -> ("States Out"=w1101:string)  [unwired: 14 in]
        n448 = Unbundle By Name(w1093) -> ("Total Array"=w1092:dbl[], "VISA Laurel Meter"=w1097:refnum<visa-resource-name>, "FrontPanel Meters 2.Cold Water\nTotal"=w1089:dbl, "FrontPanel Meters 2.Hot Water\nTotal"=w1086:dbl, "FrontPanel Meters 2.Cold Water Total During Wash"=w1061:dbl, "FrontPanel Meters 2.Hot Water Total During Wash"=w1062:dbl, "FrontPanel Meters 2.Rinse Cold"=w1065:dbl, "FrontPanel Meters 2.Rinse Hot"=w1064:dbl)
        n449 = call "Laurel Meter Serial.vi"("error in (no error)"=w1100, "VISA resource name"=w1097, "Send Command"=T16."Reading: Item 1") -> ("error out"=w1080:errorcluster, "Output"=w1083:dbl)  [unwired: 7 in]
        n450 = call "Delay mS.vi"("Error In"=w1080, "milliseconds to wait"=u32 100) -> ("Error Out"=w1079:errorcluster)  [unwired: 13 in]
        n451 = Greater?(x=w1083, y=0.0) -> (0:w1087:bool)
        n452 = case shown="True" w1087 {
          tunnel: [w1130 w1132] -> w1070
          tunnel: w1089 -> [w1130 w1133]
          tunnel: w1083 -> [_ w1137]
          tunnel: [0.0 w1135] -> w1084
          frame False {
          }
          frame True {
            n453 = local read "Elapsed Time"() -> (w1139:dbl)
            n454 = Greater?(x=w1139, y=20.0) -> (0:w1140:bool)
            n455 = case shown="True" w1140 {
              tunnel: [0.0 w1142] -> w1136
              frame False {
                # "The Laurel Meters\nhave some jitter on\ninitial startup"
              }
              frame True {
                n456 = local read "Loop Time"() -> (w1144:dbl)
                n457 = Divide(x=w1144, y=60.0) -> (x/y=w1142:dbl)
              }
            }
            n458 = call "Pulse2GPM.vi"("Pulse/Second"=w1137) -> ("GPM"=w1135:dbl)  [unwired: 10 in]
            n459 = Multiply(x=w1135, y=w1136) -> (x*y=w1134:dbl)
            n460 = Add(x=w1134, y=w1133) -> (x+y=w1132:dbl)
          }
        }
        n461 = call "Laurel Meter Serial.vi"("error in (no error)"=w1079, "VISA resource name"=w1097, "Send Command"=T16."Reading: Item 2") -> ("error out"=w1098:errorcluster, "Output"=w1082:dbl)  [unwired: 7 in]
        n462 = Greater?(x=w1082, y=0.0) -> (0:w1085:bool)
        n463 = Search 1D Array(1D array=w1075, element="Drain ON") -> (index of element=w1073:i32)  [unwired: 1 in]
        n464 = case shown="True" w1085 {
          tunnel: [0.0 w1119] -> w1081
          tunnel: w1086 -> [w1116 w1120]
          tunnel: [w1116 w1117] -> w1069
          tunnel: w1082 -> [_ w1122]
          frame False {
          }
          frame True {
            n465 = local read "Elapsed Time"() -> (w1124:dbl)
            n466 = Greater?(x=w1124, y=20.0) -> (0:w1123:bool)
            n467 = case shown="True" w1123 {
              tunnel: [0.0 w1127] -> w1118
              frame False {
                # "The Laurel Meters\nhave some jitter on\ninitial startup"
              }
              frame True {
                n468 = local read "Loop Time"() -> (w1129:dbl)
                n469 = Divide(x=w1129, y=60.0) -> (x/y=w1127:dbl)
              }
            }
            n470 = call "Pulse2GPM.vi"("Pulse/Second"=w1122) -> ("GPM"=w1119:dbl)  [unwired: 10 in]
            n471 = Multiply(x=w1119, y=w1118) -> (x*y=w1121:dbl)
            n472 = Add(x=w1121, y=w1120) -> (x+y=w1117:dbl)
          }
        }
        n473 = Equal?(x=w1073, y=-1) -> (x = y?=w1071:bool)
        n474 = case shown="False" w1071 {
          tunnel: w1070 -> [w1105 w1114]
          tunnel: w1069 -> [w1106 w1113]
          tunnel: [w1103 w1114] -> w1068
          tunnel: [w1104 w1113] -> w1067
          tunnel: w1061 -> [w1110 _]
          tunnel: [w1109 w1112] -> w1063
          tunnel: w1062 -> [w1108 _]
          tunnel: [w1107 w1111] -> w1066
          tunnel: w1065 -> [_ w1112]
          tunnel: w1064 -> [_ w1111]
          tunnel: w1062 -> [w1104 _]
          tunnel: w1061 -> [w1103 _]
          frame False {
            # "Rinse Fill Amount"
            n475 = Subtract(x=w1105, y=w1110) -> (x-y=w1109:dbl)
            n476 = Subtract(x=w1106, y=w1108) -> (x-y=w1107:dbl)
          }
          frame True {
            # "Wash Fill Amount"
          }
        }
        n477 = Build Array (concatenate)(w1092, w1084, w1070, w1081, w1069) -> (w1094:dbl[])
        n478 = Bundle By Name(cluster=w1093, "Total Array"=w1094, "FrontPanel Meters 2.Cold Water\nRate"=w1084, "FrontPanel Meters 2.Hot Water\n Rate"=w1081, "FrontPanel Meters 2.Cold Water\nTotal"=w1070, "FrontPanel Meters 2.Hot Water\nTotal"=w1069, "FrontPanel Meters 2.Cold Water Total During Wash"=w1068, "FrontPanel Meters 2.Hot Water Total During Wash"=w1067, "FrontPanel Meters 2.Rinse Cold"=w1063, "FrontPanel Meters 2.Rinse Hot"=w1066) -> (w1095:T19)
      }
      frame "Get Power Data" {
        # "This is Watt Hours"
        n479 = Unbundle By Name(w1155) -> ("Total Array"=w1153:dbl[], "Aplus IP Address"=w1160:string, "Remote Port"=w1159:i32)
        n480 = call "APLUS Camille Bauer Driver.vi"("error in (no error)"=w1158, "Remote Port"=w1159, "Remote IP Address"=w1160) -> ("error out"=w1157:errorcluster, "output cluster"=w1156:T24)  [unwired: 7 in]
        n481 = Unbundle By Name(w1156) -> ("Voltage"=w1152:sgl, "Current"=w1151:sgl, "Frequency"=w1150:sgl, "Power"=w1146:sgl, "WattHours"=w1147:sgl)
        n482 = Build Array (concatenate)(w1153, w1152, w1151, w1150, w1146, w1147) -> (w1149:dbl[])
        n483 = Bundle By Name(cluster=w1155, "Total Array"=w1149, "FrontPanel Meters 2.Volts"=w1152, "FrontPanel Meters 2.Current"=w1151, "FrontPanel Meters 2.Watts"=w1146, "FrontPanel Meters 2.Watt Hour"=w1147) -> (w1154:T19)
        n484 = call <vilib>:"Add State(s) to Queue__jki_lib_state_machine.vi"("State(s) in (\"\")"=w1162) -> ("States Out"=w1161:string)  [unwired: 14 in]
      }
      frame "Check Newfi" {
        # "This is Watt Hours"
        n485 = Unbundle By Name(w1175) -> ("Total Array"=w1174:dbl[])
        n486 = local read "Drain"() -> (w1201:bool)
        n487 = local read "FS"() -> (w1177:bool)
        n488 = local read "Lid Closed?"() -> (w1195:bool)
        n489 = local read "Lid Locked?"() -> (w1193:bool)
        n490 = local read "Cold"() -> (w1203:bool)
        n491 = local read "Hot"() -> (w1205:bool)
        n492 = local read "Recirc"() -> (w1198:bool)
        n493 = case shown="False" w1177 {
          tunnel: ["Fabric Softener OFF" "Fabric Softener ON"] -> w1176
          frame False {
          }
          frame True {
          }
        }
        n494 = local read "Det"() -> (w1197:bool)
        n495 = case shown="True" w1205 {
          tunnel: ["Hot OFF" "Hot ON"] -> w1204
          frame False {
          }
          frame True {
          }
        }
        n496 = case shown="False" w1203 {
          tunnel: ["Cold OFF" "Cold ON"] -> w1202
          frame False {
          }
          frame True {
          }
        }
        n497 = case shown="True" w1201 {
          tunnel: ["Drain OFF" "Drain ON"] -> w1200
          frame False {
          }
          frame True {
          }
        }
        n498 = case shown="False" w1198 {
          tunnel: ["Recirc Pump OFF" "Recirc Pump ON"] -> w1199
          frame False {
          }
          frame True {
          }
        }
        n499 = case shown="False" w1193 {
          tunnel: ["Lid Unlocked" "Lid Locked"] -> w1192
          frame False {
          }
          frame True {
          }
        }
        n500 = case shown="True" w1197 {
          tunnel: ["Detergent OFF" "Detergent ON"] -> w1196
          frame False {
          }
          frame True {
          }
        }
        n501 = case shown="True" w1195 {
          tunnel: ["Lid Open" "Lid Closed"] -> w1194
          frame False {
          }
          frame True {
          }
        }
        n502 = local read "Fabric Softener"() -> (w1187:u32)
        n503 = local read "Temperature"() -> (w1191:u8)
        n504 = local read "Detergent"() -> (w1189:u32)
        n505 = local read "Load Size"() -> (w1190:u32)
        n506 = for {
          tunnel: w1174 -> [w1216] mode=indexing
          tunnel: [w1215] -> w1173 mode=indexing
          n507 = Number To Fractional String(number=w1216, precision (6)=i16 3) -> (F-format string=w1215:string)  [unwired: 2 in]
        }
        n508 = local read "Direction"() -> (w1171:string)
        n509 = local read "Speed"() -> (w1186:u32)
        n510 = local read "Water Pressure"() -> (w1188:u32)
        n511 = Number To Decimal String(number=w1191) -> (decimal integer string=w1185:string)  [unwired: 1 in]
        n512 = Number To Decimal String(number=w1190) -> (decimal integer string=w1184:string)  [unwired: 1 in]
        n513 = Number To Decimal String(number=w1189) -> (decimal integer string=w1183:string)  [unwired: 1 in]
        n514 = Number To Decimal String(number=w1187) -> (decimal integer string=w1182:string)  [unwired: 1 in]
        n515 = Number To Decimal String(number=w1186) -> (decimal integer string=w1180:string)  [unwired: 1 in]
        n516 = Number To Decimal String(number=w1188) -> (decimal integer string=w1181:string)  [unwired: 1 in]
        n517 = Build Array(w1204, w1202, w1200, w1176, w1199, w1196, w1194, w1192, w1185, w1184, w1183, w1182, w1181, w1180, w1171) -> (w1170:string[])
        n518 = call <vilib>:"Add State(s) to Queue__jki_lib_state_machine.vi"("State(s) in (\"\")"=w1209) -> ("States Out"=w1208:string)  [unwired: 14 in]
        n519 = Get Date/Time In Seconds() -> (seconds since 1Jan1904=w1169:timestamp)
        n520 = Get Date/Time String(seconds (now)=w1169) -> (date string=w1168:string, time string=w1164:string)  [unwired: 2 in]
        n521 = for {
          N: 2 -> [_]
          shift-right: [w1210] -> w1166
          shift-left: w1168 -> [w1213]
          n522 = Search and Replace String(input string=w1213, search string="/", replace string="-" ("replace string (\"\")")) -> (result string=w1210:string)  [unwired: 5 in, 3 out]
        }
        n523 = call <vilib>:"Space Constant.vi"() -> ("String"=w1163:string)
        n524 = Concatenate Strings(w1166, w1163, w1164) -> (w1165:string)
        n525 = Build Array (concatenate)(w1165, w1173, w1170) -> (w1172:string[])
        n526 = Build Array (concatenate)(w1179, w1172) -> (w1178:string[][])
      }
      frame "Show Data" {
        n527 = Unbundle By Name(w1238) -> ("FrontPanel Meters 2"=→"FrontPanel Meters":T1, "Total Array"=w1241:dbl[], "First Time Through"=w1239:bool, "Calibration"=w1234:string[][], "FrontPanel Meters 2.Watts"=→"Recirc 3":dbl)
        n528 = Build Array (concatenate)(w1243, w1241) -> (w1242:dbl[][])
        n529 = call <vilib>:"Add State(s) to Queue__jki_lib_state_machine.vi"("State(s) in (\"\")"=w1247) -> ("States Out"=w1246:string)  [unwired: 14 in]
        n530 = case shown="True" w1239 {
          tunnel: w1240 -> [w1249 w1256]
          tunnel: [w1249 w1250] -> w1235
          tunnel: [FALSE FALSE] -> w1236
          tunnel: w1234 -> [_ w1252]
          frame False {
          }
          frame True {
            n531 = Insert Into Array(array=w1256, index (row)=0, new element=string[] ["Date", "Time (Seconds)\nTime (Seconds)\nTime (Seconds)\n", "Cold Water Pressure (PSI)\n", "Hot Water Pressure (PSI)\n", "Cold Water Temp (F)\n", "Hot Water Temp (F)\n", "Ambient Temp (F)\n", "RH (%)\n", "Cold Water Rate (GPM)\n", "Cold Water Total (Gal)\n", "Hot Water Rate (GPM)\n", "Hot Water Total (Gal)\n", "Voltage\n", "Current\n", "Frequency\n", "Watts\n", "Watt Hours\n", "Hot Water Valve\n", "Cold Water Valve\n", "Drain Valve\n", "Fabric Softener Pump", "Recirc Pump\n", "Detergent Pump\n", "Lid Status\n", "Lid Lock\n", "Temperature\n", "Load Size\n", "Detergent\n", "Fabric Softener\n", "Water Pressure\n", "Speed (RPM)\n", "Direction\n"]) -> (w1253:string[][])  [unwired: 1 in]
            n532 = Insert Into Array(array=w1253, index (row)=0, new element=w1252) -> (w1250:string[][])  [unwired: 1 in]
          }
        }
        "Array" <- w1235
        n533 = Bundle By Name(cluster=w1238, "First Time Through"=w1236) -> (w1237:T19)
      }
    }
  }
